vi "MHM_DLLDemo.vi"() -> ()   [LabVIEW 2019]
uses:
  enums/MHM_ConfigDataEnum.ctl
  enums/MHM_InterfaceEnum.ctl
  enums/MHM_ParamEnum.ctl
  enums/MHM_WriteVerifyEnum.ctl
  enums/EdsParamEnum.ctl
  enums/MHM_E2PRangeEnum.ctl
  enums/MHM_CalDataEnum.ctl
  enums/MHM_CalParamEnum.ctl
  enums/MHM_ErrorTypeEnum.ctl
  enums/MHM_CalCfgEnum.ctl
  enums/MHM_InterfaceInfoEnum.ctl
  MHM_1SL_interface.lvlib
panel:
  in  "StopButton":bool
  out "running":bool
  in  "TabControl":T1(tab)
  in  "MHM_InterfaceInfoEnum":T2
  out "MHM_InterfaceEnum":T3
  in  "MHM_InterfaceEnum":T3
  out "InterfaceLED":bool
  out "OpenLED":bool
  in  "MHM_Close":bool
  in  "MHM_GetInterface":bool
  in  "MHM_SetInterface":bool
  in  "MHM_Open":bool
  in  "pcInterfaceOption":string
  in  "MHM_GetInterfaceInfo":bool
  out "pcInterfaceInfo":string
  in  "MHM_Initialize":bool
  out "pulValue":u32 format="0x%02x"
  in  "ulValue":u32 format="0x%02x"
  in  "MHM_ConfigEnum":T4
  in  "MHM_ConfigEnum":T4
  in  "MHM_GetConfig":bool
  in  "MHM_SetConfig":bool
  in  "MHM_SwitchToBiSS":bool
  out "pulEnSsi":u32 format="0x%02x"
  in  "MHM_E2PRangeEnum":T5
  in  "MHM_WriteEeprom":bool
  in  "MHM_ReadStatusRegister":bool
  in  "ulWriteVerify":u32 format="0x%02x"
  in  "ulValue SetParam":u32 caption="ulValue" format="0x%02x"
  out "ulValue GetParam":u32 caption="pulValue" format="0x%02x"
  in  "MHM_WriteVerifyEnum":T6
  in  "MHM_ParamEnum":T7
  in  "MHM_ParamEnum":T7
  in  "MHM_WriteParams":bool
  in  "MHM_SetParam":bool
  in  "MHM_GetParam":bool
  in  "MHM_ReadParams":bool
  in  "MHM_ReadEeprom":bool
  in  "MHM_E2PRangeEnum":T5
  out "pulValid":u32[](array[numeric]) format="0x%02x"
  in  "MHM_GetCorrectedRegisters":bool
  out "pulCorrected":u32[](array[numeric]) format="0x%02x"
  in  "MHM_ReadGainRegister":bool
  in  "MHM_ReadSens":bool
  out "pulGain":u32 format="0x%02x"
  out "pSensorDataStruct":T8 {"pulGainRegister" format="0x%02x"; "pulPortRegister" format="0x%02x"; "pulStatusRegister" format="0x%02x"; "pulLifecounter" format="0x%02x"; "pulWarning" format="0x%02x"; "pulError" format="0x%02x"; "pulSingleturn" format="0x%02x"; "pulMultiturn" format="0x%02x"; "pulDataLength" format="0x%02x"; "pulLowData" format="0x%02x"; "pulHighData" format="0x%02x"}
  in  "MHM_CalParamEnum":T9
  in  "pulNumberOfBytes":u32 format="0x%02x"
  in  "ulCycles":u32=4096 format="0x%02x"
  in  "MHM_FullAcquisition":bool
  in  "ulCycles":u32=4096 format="0x%02x"
  in  "MHM_FullCalibration":bool
  in  "MHM_GetCalData":bool
  in  "MHM_GetCalParam":bool
  in  "MHM_CalDataEnum":T10
  out "plData":i32[](array[numeric]) format="0x%02x"
  out "plData":i32 format="0x%02x"
  in  "MHM_SetCalCfg":bool
  in  "MHM_CalCfgEnum":T11
  in  "lValue":i32 format="0x%02x"
  in  "MHM_CalCfgEnum":T11
  in  "MHM_GetCalCfg":bool
  out "plValue":i32 format="0x%02x"
  in  "MHM_SetCalData":bool
  in  "ulNumberOfBytes":u32 format="0x%02x"
  in  "MHM_CalDataEnum":T10
  in  "plData":i32[](array[numeric]) format="0x%02x"
  in  "MHM_AdjustGain":bool
  in  "MHM_ActivateCalCfg":bool
  in  "MHM_AcquireEx":bool
  in  "ulCycles":u32 format="0x%02x"
  in  "MHM_DeactivateCalCfg":bool
  in  "MHM_AnalyzeData":bool
  in  "MHM_Adjust":bool
  in  "MHM_WriteVerifyEnum":T6
  out "pulValue 2":u32 caption="pulValue" format="0x%02x"
  in  "ulValue":u32 format="0x%02x"
  in  "EdsParamEnum":T12 caption="MHM_EdsParamEnum"
  in  "MHM_EdsParamEnum":T12
  in  "MHM_SetEdsParam":bool
  in  "MHM_GetEdsParam":bool
  in  "MHM_ReadEdsParams":bool
  in  "MHM_UpdateEds":bool
  in  "ulCommand":u32=1 min=1 max=2 format="0x%02x"
  in  "MHM_ReadPorts":bool
  in  "MHM_WritePorts":bool
  in  "MHM_WriteCommand":bool
  in  "MHM_SPIActivate":bool
  in  "MHM_GetDLLVersion":bool
  in  "MHM_SaveParams":bool
  in  "MHM_LoadParams":bool
  in  "pcFilename":string
  in  "pcFilename":string
  out "pulDllVersion":u32[](array[numeric]) format="0x%02x"
  in  "ulPorts":u32 format="0x%02x"
  out "pulPorts":u32 format="0x%02x"
  in  "ulData":u32 format="0x%02x"
  in  "MHM_GetLastError":bool
  out "pulLastError":u32 format="0x%02x"
  out "MHM_ErrorTypeEnum":T13
  out "pcErrorText":string
  in  "MHM_Preset":bool
  in  "MHM_LoadRegister":bool
  in  "MHM_SaveRegister":bool
  in  "MHM_ReadRegister":bool
  in  "MHM_WriteRegister":bool
  in  "MHM_GetRegister":bool
  in  "MHM_SetRegister":bool
  in  "ulAdr":u32 format="0x%02x"
  in  "ulValue 2":u32 caption="ulValue" format="0x%02x"
  in  "MHM_WriteVerifyEnum 2":T6 caption="MHM_WriteVerifyEnum"
  in  "ulAdr":u32 format="0x%02x"
  out "pulValue":u32 format="0x%02x"
  in  "ulAdr 3":u32 caption="ulAdr" format="0x%02x"
  in  "pulNumberOfBytes":u32 format="0x%02x"
  in  "pulData":u32[](array[numeric]) format="0x%02x"
  out "pulData":u32[](array[numeric]) format="0x%02x"
  in  "pulNumberOfBytes":u32 format="0x%02x"
  in  "ulAdr":u32 format="0x%02x"
  in  "pcFilename 3":string caption="pcFilename"
  in  "ulAdr 5":u32 caption="ulAdr" format="0x%02x"
  in  "pulData 3":u32[](array[numeric]) caption="pulData" format="0x%02x"
  in  "pulNumberOfBytes5":u32 caption="pulNumberOfBytes" format="0x%02x"
  in  "pcFilename":string
  in  "ulAdr":u32 format="0x%02x"
  out "pulData":u32[](array[numeric]) format="0x%02x"
  in  "pulNumerOfBytes":u32 format="0x%02x"
  in  "MHM_WriteRegister_I2C":bool
  in  "ulAdr":u32 format="0x%02x"
  in  "ulNumberOfBytes":u32 format="0x%02x"
  in  "ulI2CSlaveAdr":u32 format="0x%02x"
  in  "pulData":u32[](array[numeric]) format="0x%02x"
  in  "MHM_ReadRegister_I2C":bool
  in  "ulAdr":u32 format="0x%02x"
  in  "pulNumberOfBytes":u32 format="0x%02x"
  in  "ulI2CSlaveAdr":u32 format="0x%02x"
  out "pulData":u32[](array[numeric]) format="0x%02x"
  in  "MHM_WriteRegister_I2C_EX":bool
  in  "ulArraySize":u32 format="0x%02x"
  in  "ulI2CSlaveAdr":u32 format="0x%02x"
  in  "pulData":u32[](array[numeric]) format="0x%02x"
  in  "pulValid":u32[](array[numeric]) format="0x%02x"
  in  "MHM_LoadRegister_EX":bool
  in  "pcFilename":string
  in  "ulArraySize":u32=256 format="0x%02x"
  out "pulData":u32[](array[numeric]) format="0x%02x"
  out "pulValid":u32[](array[numeric]) format="0x%02x"
  in  "MHM_SaveRegister_EX":bool
  in  "pcFilename":string
  in  "ulAdr":u32 format="0x%02x"
  in  "pulNumberOfBytes":u32 format="0x%02x"
  in  "pulData":u32[](array[numeric]) format="0x%02x"
  # "MHM_DLLDemo"
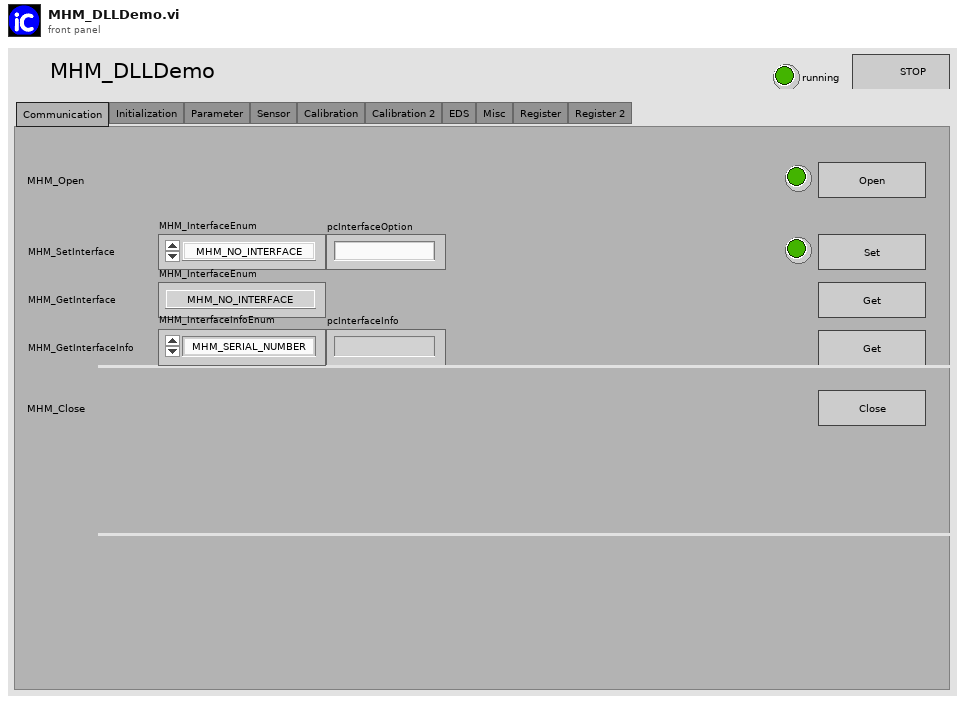
[diagram p1: front panel]
types:
  T1 = enum32{"Communication", "Initialization", "Parameter", "Sensor", "Calibration", "Calibration 2", "EDS", "Misc", "Register", "Register 2"}
  T2 = typedef "MHM_InterfaceInfoEnum.ctl" = enum16{"MHM_SERIAL_NUMBER"}
  T3 = typedef "MHM_InterfaceEnum.ctl" = enum16{"MHM_NO_INTERFACE", "MHM_MB3U_SPI", "MHM_MB3U_BISS", "MHM_MB4U", "MHM_MB5U"}
  T4 = typedef "MHM_ConfigDataEnum.ctl" = enum16{"MHM_CHIPVERSION", "MHM_USEUSB", "MHM_USELPT", "MHM_MASTERVER", "MHM_MASTERREV", "MHM_SLAVE_ID", "MHM_SLAVECOUNT", "MHM_FREQ_SCD", "MHM_FREQ_AGS", "MHM_FREQ_SPI", "MHM_CLKENI", "MHM_BP", "MHM_MT_TYPE", "MHM_RESERVED0", "MHM_RESERVED1", "MHM_RESERVED2", "MHM_RESERVED3", "MHM_FREQ_SSI", "MHM_READ_STATUS_ENABLE", "MHM_READ_PORTS_ENABLE", "MHM_READ_GAIN_ENABLE", "MHM_USB_PERFORMANCE", "MHM_ENABLE_TTL", "MHM_UPDATE_BISSID_ENABLE", "eMHM_DISABLE_AUTOMATIC_TTL_SWITCH"}
  T5 = typedef "MHM_E2PRangeEnum.ctl" = enum16{"MHM_E2P_CFG_MHM", "MHM_E2P_CFG_MT", "MHM_E2P_EDS", "MHM_E2P_ALL", "MHM_E2P_CFG_MHM_NO_OFFS"}
  T6 = typedef "MHM_WriteVerifyEnum.ctl" = enum16{"MHM_SETONLY", "MHM_WRITE", "MHM_VERIFY"}
  T7 = typedef "MHM_ParamEnum.ctl" = enum16{"MHM_AVGFILT", "MHM_TLF", "MHM_DIR", "MHM_HYS", "MHM_RESO_MT", "MHM_RESO_ST", "MHM_CF_MTI", "MHM_SBL_MTI", "MHM_EBL_MTI", "MHM_GET_MTI", "MHM_CFG_IOP", "MHM_MT12", "MHM_RTX_MODE", "MHM_BIN_SSI", "MHM_EXT_SSI", "MHM_ENSSI", "MHM_VOSS", "MHM_VOSC", "MHM_CIBM", "MHM_ENF", "MHM_TEST", "MHM_GAINF", "MHM_GAINR", "MHM_GCC", "MHM_ENAC", "MHM_CRCS", "MHM_ENLC", "MHM_REGPROT", "MHM_INSPROT", "MHM_PRES_IO1", "MHM_DIR_IO2", "MHM_ENCMD3", "MHM_ENCMD2", "MHM_CRC_CFG", "MHM_OFFS_MT", "MHM_OFFS_ST", "MHM_CRC_OFFS", "MHM_PSET_MT", "MHM_PSET_ST", "MHM_CRC_PSET", "MHM_ERR_CFG", "MHM_ERR_OFFS", "MHM_ERR_POS", "MHM_ERR_EXT", "MHM_ERR_AMIN", "MHM_ERR_AMAX", "MHM_ERR_MTI", "MHM_ERR_MT", "MHM_GAIN", "MHM_EDSBANK", "MHM_PRO_ID", "MHM_DEV_ID0", "MHM_DEV_ID1", "MHM_DEV_ID2", "MHM_DEV_ID3", "MHM_DEV_ID4", "MHM_DEV_ID5", "MHM_MFG_ID0", "MHM_MFG_ID1", "MHM_HARMCAL", "MHM_DISBISS", "MHM_NTOA", "MHM_ENCMD01", "MHM_CHIP_REL"}
  T8 = cluster{"pulHighData":u32, "pulLowData":u32, "pulDataLength":u32, "pulMultiturn":u32, "pulSingleturn":u32, "pulError":u32, "pulWarning":u32, "pulLifecounter":u32, "pulStatusRegister":u32, "pulPortRegister":u32, "pulGainRegister":u32}
  T9 = typedef "MHM_CalParamEnum.ctl" = enum16{"MHM_CAL_SINOFF", "MHM_CAL_COSOFF", "MHM_CAL_GAINCOSCORR", "MHM_CAL_HARM4", "MHM_CAL_RPM"}
  T10 = typedef "MHM_CalDataEnum.ctl" = enum16{"MHM_DUTRAW", "MHM_DUTCONT", "MHM_REFCONT", "MHM_DUTERR", "MHM_ADJERR", "MHM_REFRAW"}
  T11 = typedef "MHM_CalCfgEnum.ctl" = enum16{"MHM_CAL_FREQ_SPI", "MHM_CAL_FREQ_SCD", "MHM_CAL_FREQ_AGS", "MHM_CAL_REF_TYPE", "MHM_CAL_REF_RES", "MHM_CAL_REF_PER", "MHM_CAL_QUALITY_CHECK"}
  T12 = typedef "EdsParamEnum.ctl" = enum16{"EDS_EDS_VER", "EDS_EDS_LEN", "EDS_USR_STA", "EDS_USR_END", "EDS_TMA", "EDS_TO_MIN", "EDS_TO_MAX", "EDS_TOS_MIN", "EDS_TOS_MAX", "EDS_TCLK_MIN", "EDS_TCLK_MAX", "EDS_TCYC", "EDS_TBUSY_S", "EDS_BUSY_S", "EDS_PON_DLY", "EDS_DC_NUM", "EDS_SL_NUM", "EDS_SL_OFF", "EDS_BANK1", "EDS_DLEN1", "EDS_FORMAT1_STOP", "EDS_FORMAT1_ALIGN", "EDS_FORMAT1_TYPE", "EDS_CPOLY1", "EDS_BANK2", "EDS_DLEN2", "EDS_FORMAT2_STOP", "EDS_FORMAT2_ALIGN", "EDS_FORMAT2_TYPE", "EDS_CPOLY2", "EDS_BANK3", "EDS_DLEN3", "EDS_FORMAT3_STOP", "EDS_FORMAT3_ALIGN", "EDS_FORMAT3_TYPE", "EDS_CPOLY3", "EDS_BANK4", "EDS_DLEN4", "EDS_FORMAT4_STOP", "EDS_FORMAT4_ALIGN", "EDS_FORMAT4_TYPE", "EDS_CPOLY4", "EDS_BANK5", "EDS_DLEN5", "EDS_FORMAT5_STOP", "EDS_FORMAT5_ALIGN", "EDS_FORMAT5_TYPE", "EDS_CPOLY5", "EDS_BANK6", "EDS_DLEN6", "EDS_FORMAT6_STOP", "EDS_FORMAT6_ALIGN", "EDS_FORMAT6_TYPE", "EDS_CPOLY6", "EDS_BANK7", "EDS_DLEN7", "EDS_FORMAT7_STOP", "EDS_FORMAT7_ALIGN", "EDS_FORMAT7_TYPE", "EDS_CPOLY7", "EDS_BANK8", "EDS_DLEN8", "EDS_FORMAT8_STOP", "EDS_FORMAT8_ALIGN", "EDS_FORMAT8_TYPE", "EDS_CPOLY8", "EDS_BC_OFF", "EDS_BP_VER", "EDS_BP_LEN", "EDS_BP_ID", "EDS_FB1", "EDS_FB2", "EDS_PON_PDL", "EDS_EN_TYP", "EDS_POS_NUM", "EDS_MT_LEN", "EDS_MT_FMT", "EDS_CO_LEN", "EDS_CO_FMT", "EDS_FI_LEN", "EDS_FI_FMT", "EDS_MT_CNT", "EDS_SIP_CNT", "EDS_SIP_RES", "EDS_CPOLY", "EDS_CSTART", "EDS_ABS_ACU", "EDS_REL_ACU", "EDS_SPD_ACU", "EDS_HYST", "EDS_SPD_MAX", "EDS_ACC_MAX", "EDS_TMP_MIN", "EDS_TMP_MAX", "EDS_VLT_MIN", "EDS_VLT_MAX", "EDS_CUR_MAX"}
  T13 = typedef "MHM_ErrorTypeEnum.ctl" = enum16{"MHM_NONE", "MHM_HINT", "MHM_WARNING", "MHM_PROGRAMMING_ERROR", "MHM_OPERATING_ERROR", "MHM_COMMUNICATION_ERROR"}
  T14 = cluster{"ulHighData":u32, "ulLowData":u32, "ulDataLength":u32, "ulMultiturn":u32, "ulSingleturn":u32, "ulError":u32, "ulWarning":u32, "ulLifecounter":u32, "ulStatusRegister":u32, "ulPortRegister":u32, "ulGainRegister":u32}
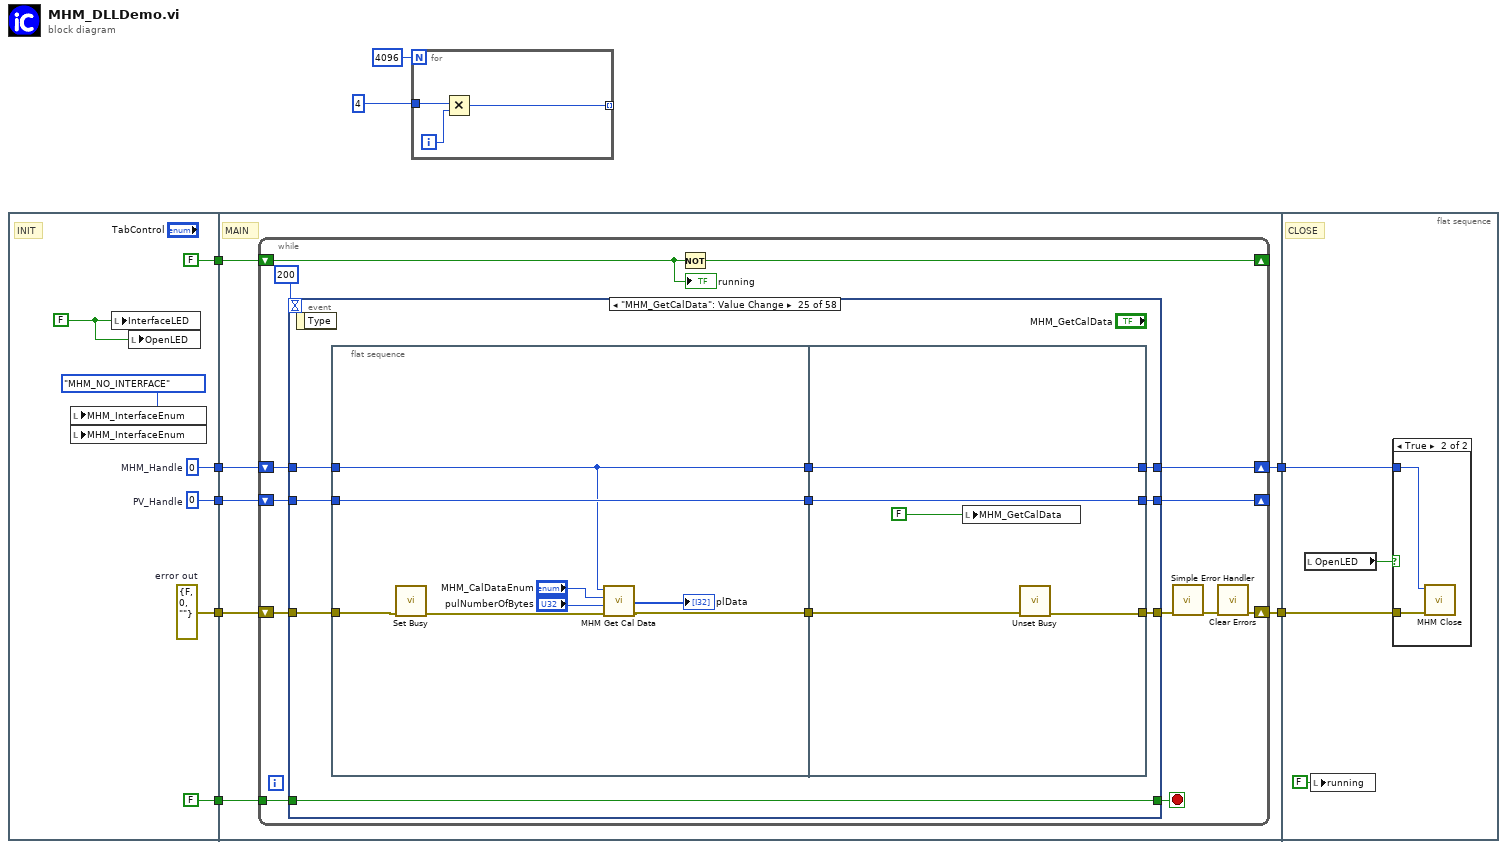
[diagram p0: block diagram]
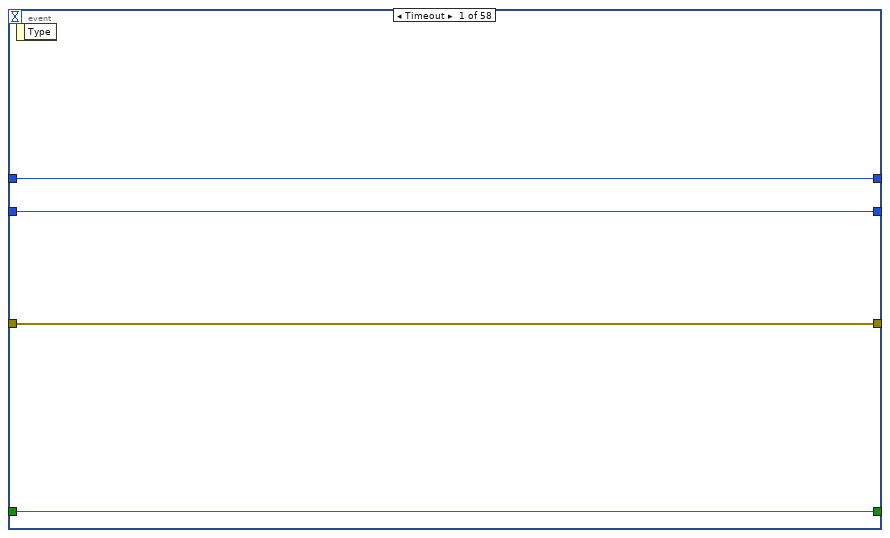
[diagram p2: hidden frame]
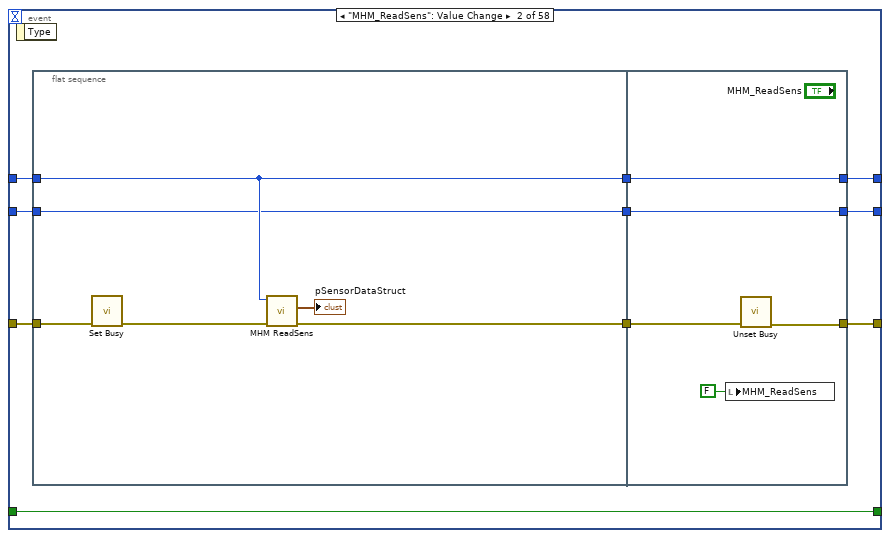
[diagram p3: hidden frame]
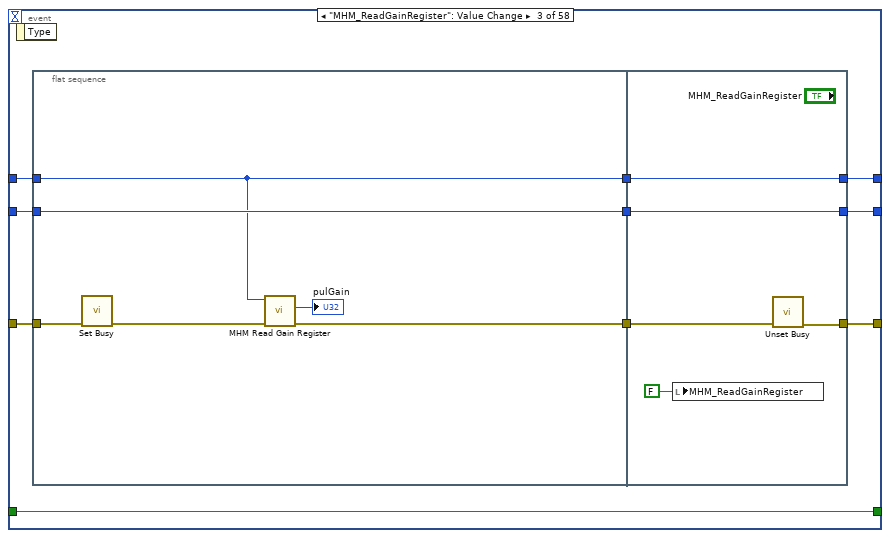
[diagram p4: hidden frame]
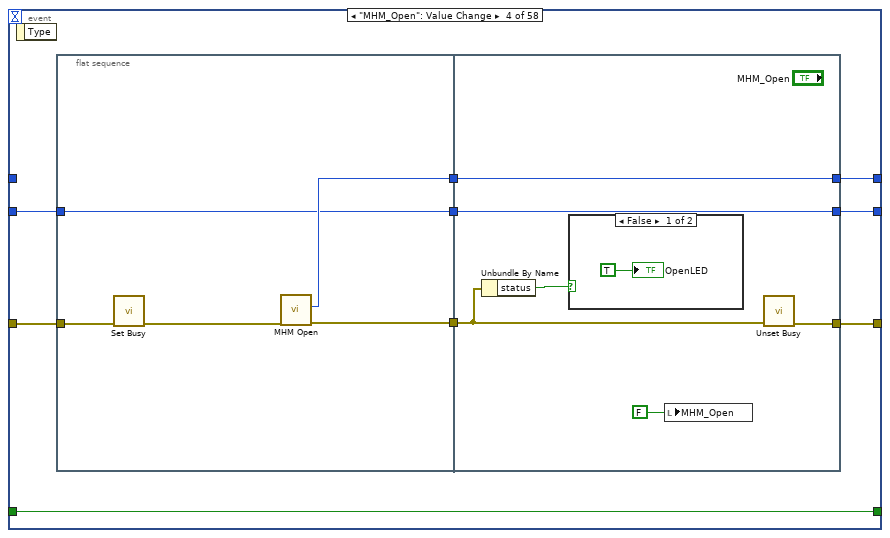
[diagram p5: hidden frame]
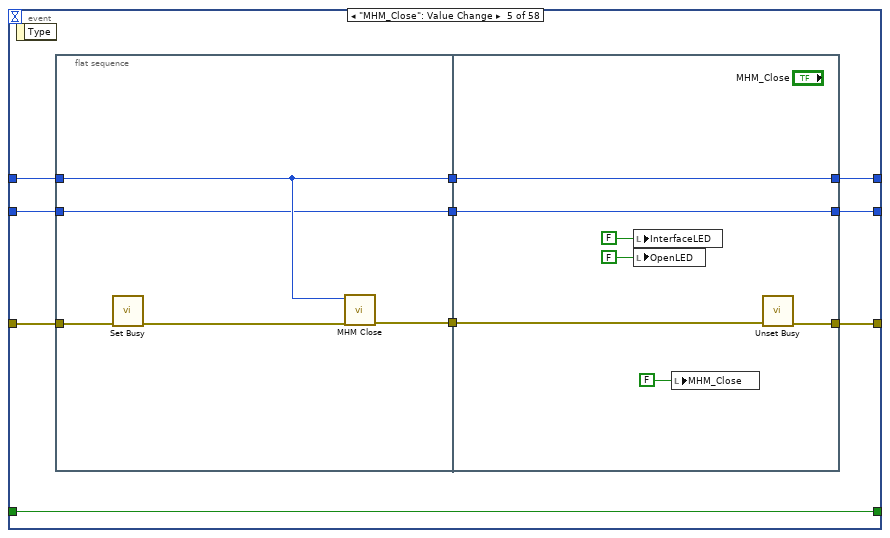
[diagram p7: hidden frame]
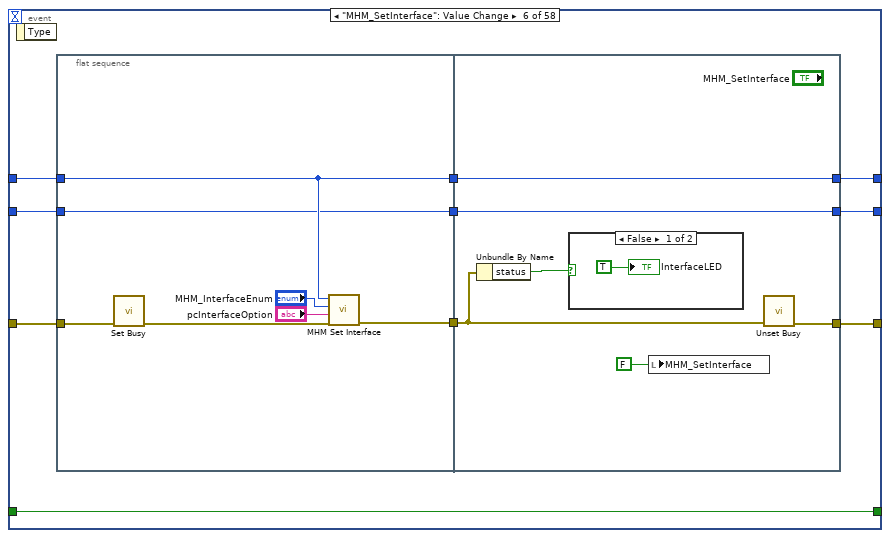
[diagram p8: hidden frame]
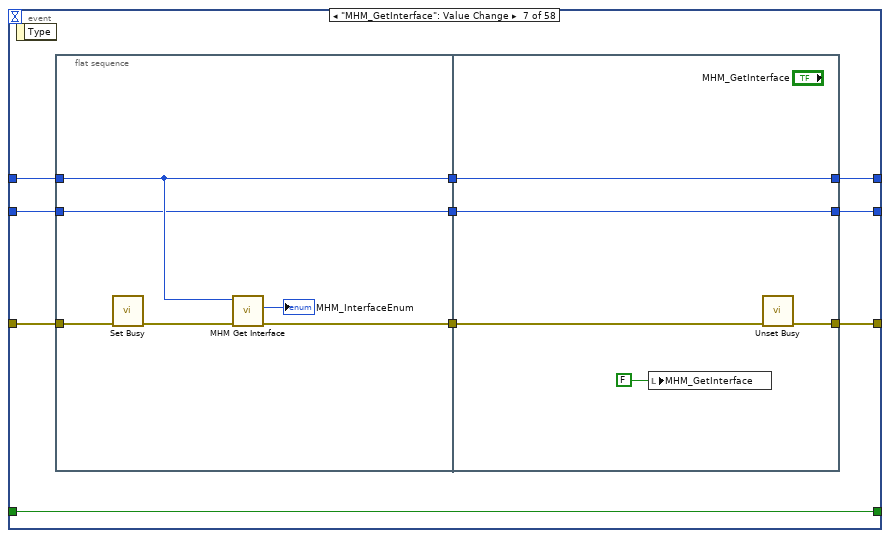
[diagram p10: hidden frame]
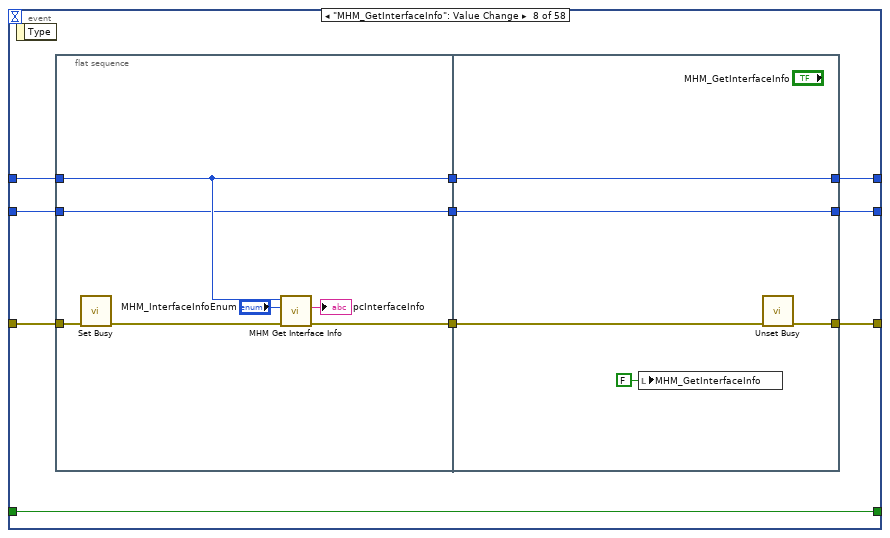
[diagram p11: hidden frame]
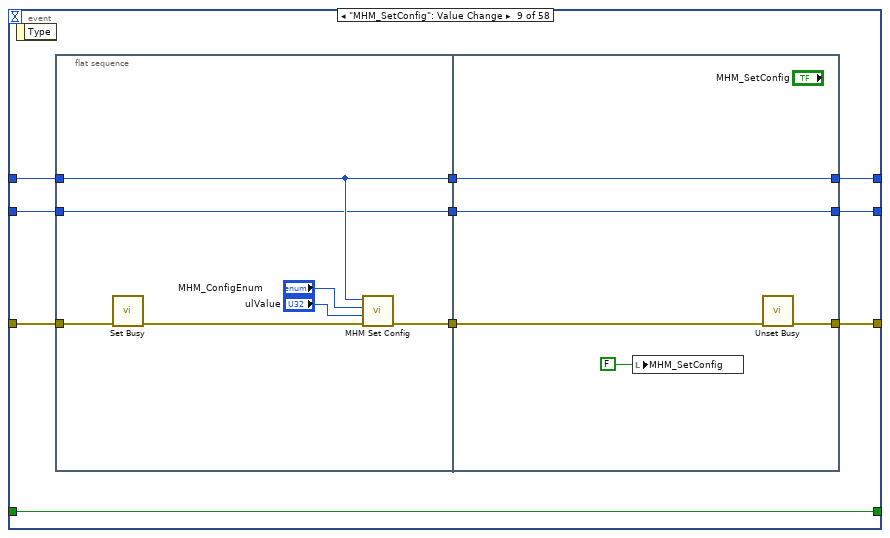
[diagram p12: hidden frame]
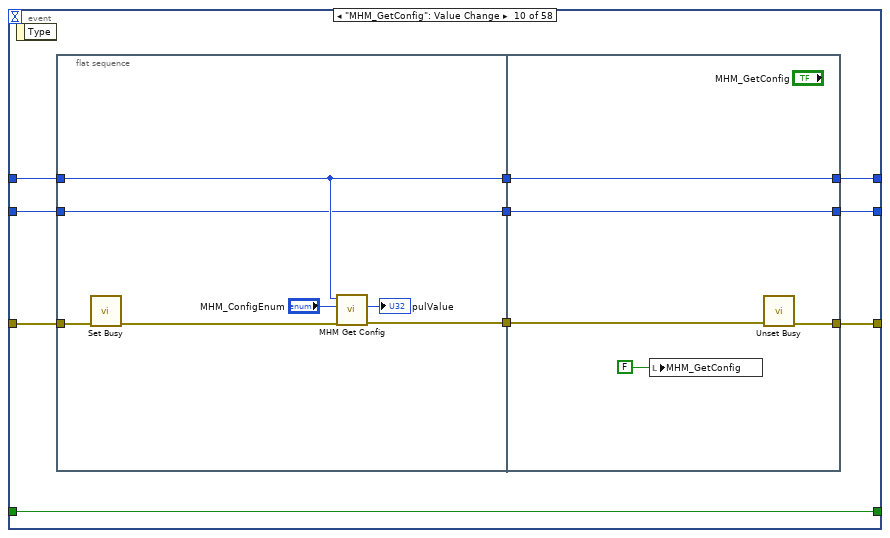
[diagram p13: hidden frame]
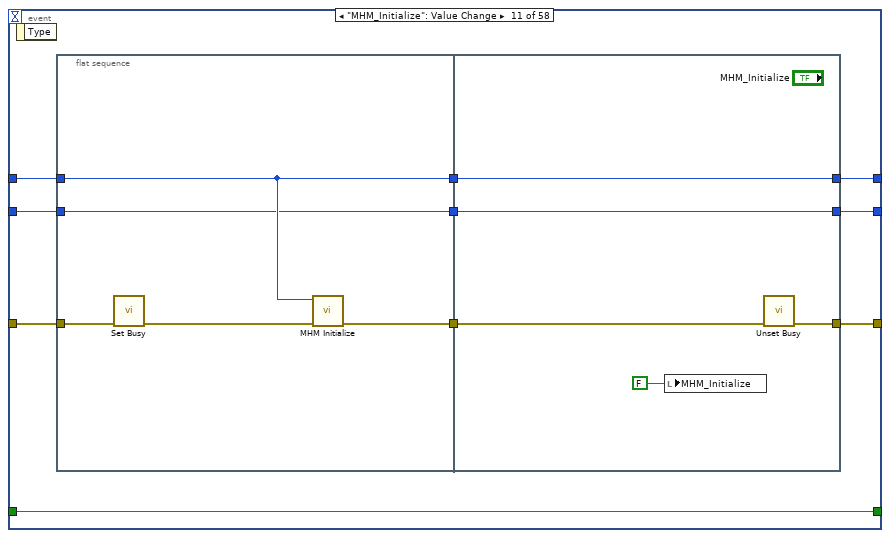
[diagram p14: hidden frame]
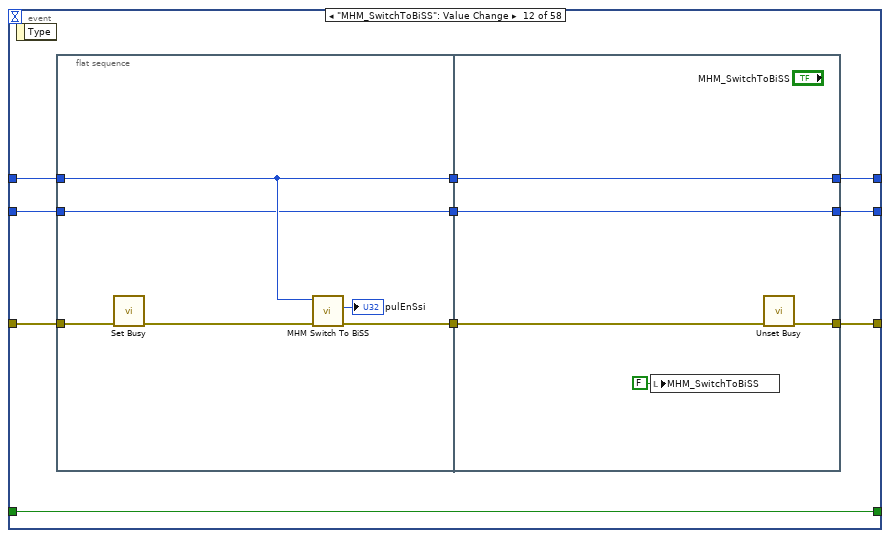
[diagram p15: hidden frame]
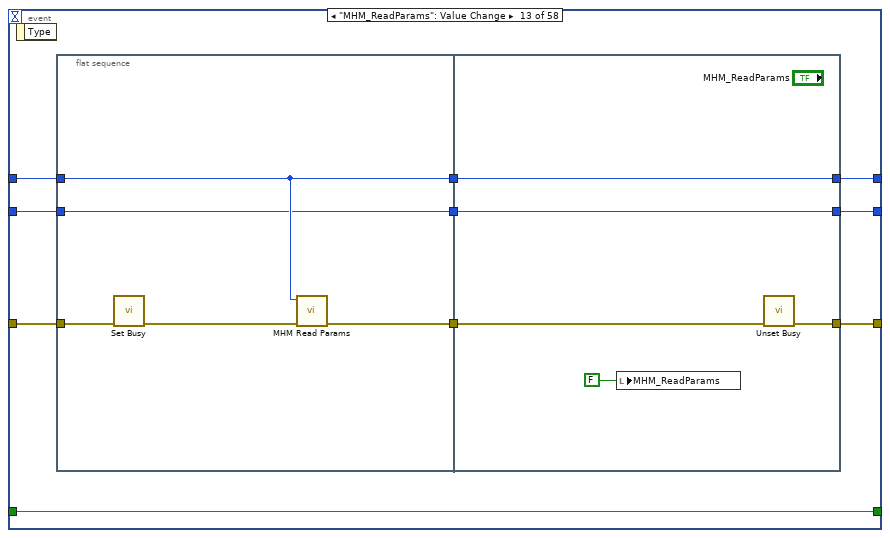
[diagram p16: hidden frame]
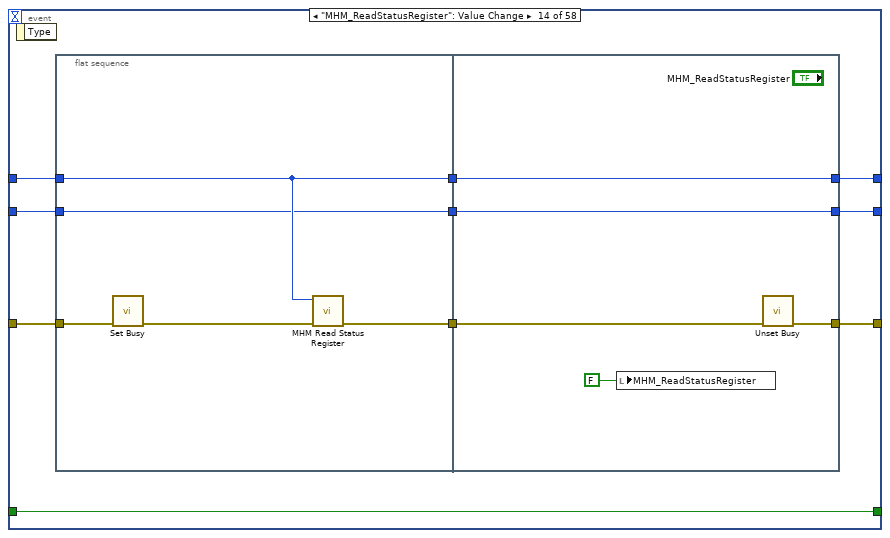
[diagram p17: hidden frame]
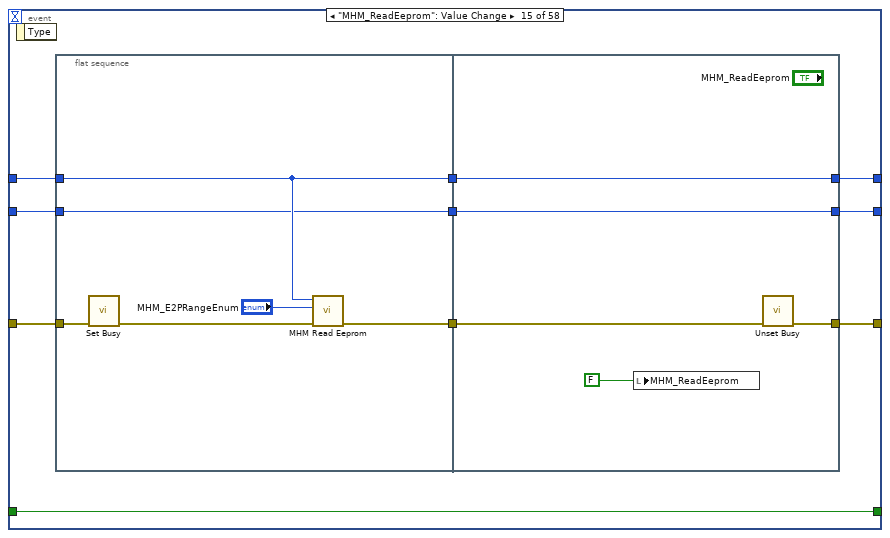
[diagram p18: hidden frame]
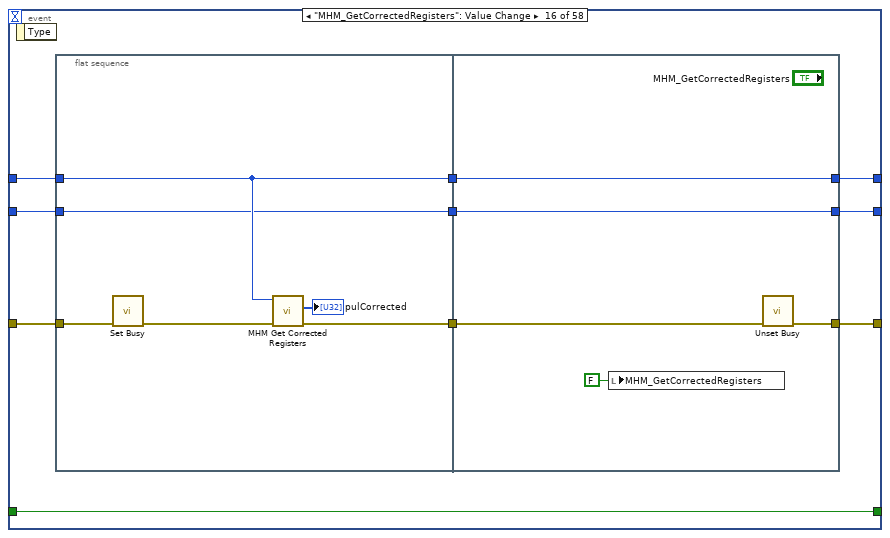
[diagram p19: hidden frame]
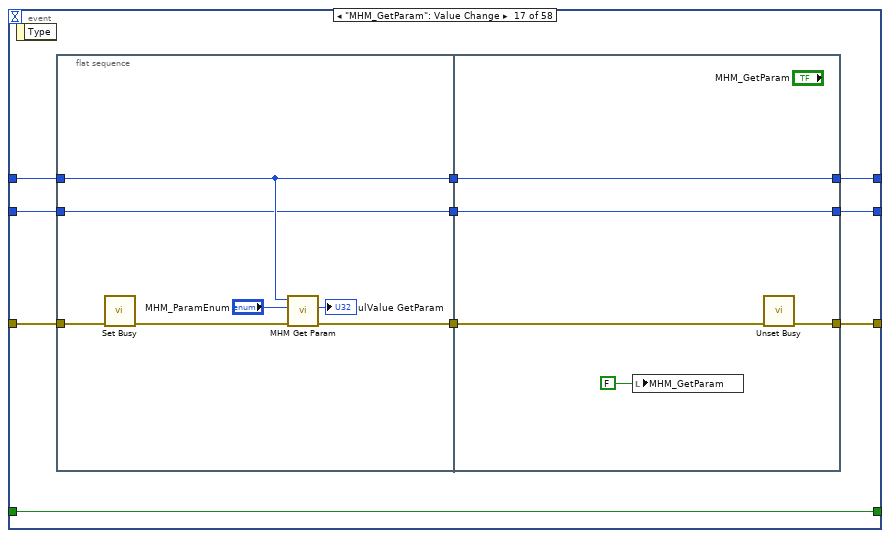
[diagram p20: hidden frame]
diagram:
  n1 = flat-sequence {
    tunnel: [FALSE] -> w9
    tunnel: [FALSE] -> w8
    tunnel: [w14] -> w7
    tunnel: [w13] -> w6
    tunnel: [w11] -> w3
    tunnel: w9 -> [w23]
    tunnel: w8 -> [w22]
    tunnel: w7 -> [w21]
    tunnel: w6 -> [w20]
    tunnel: [w19] -> w5
    tunnel: [w18] -> w4
    tunnel: w3 -> [w17]
    tunnel: w5 -> [w1263]
    tunnel: w4 -> [w1262]
    frame #0 {
      w11 = u32 0  # PV_Handle
      w12 = MHM_InterfaceEnum."MHM_NO_INTERFACE" ("MHM_InterfaceEnum")
      w10 = FALSE ("InterfaceLED")
      w13 = errorcluster {"status"=FALSE, "code"=0, "source"=""}  # error out
      w14 = u32 0  # MHM_Handle
      # "INIT"
      n2 = local write "MHM_InterfaceEnum"(w12) -> ()
      n3 = local write "MHM_InterfaceEnum"(w12) -> ()
      n4 = local write "InterfaceLED"(w10) -> ()
      n5 = local write "OpenLED"(w10) -> ()
    }
    frame #1 {
      # "MAIN"
      n6 = while {
        shift-right: [w36] -> _
        shift-left: w23 -> [w35]
        tunnel: w22 -> [w34]
        shift-right: [w27] -> w18
        shift-left: w21 -> [w32]
        shift-right: [w30] -> w19
        shift-left: w20 -> [w31]
        shift-right: [w25] -> _
        shift-left: w17 -> [w24]
        stop <- w33 stop-if-true
        n7 = event shown="[24] \"MHM_GetCalData\": Value Change" {
          selector: _ -> [_ _ _ _ _ _ _ _ _ _ _ _ _ _ _ _ _ _ _ _ _ _ _ _ _ _ _ _ _ _ _ _ _ _ _ _ _ _ _ _ _ _ _ _ _ _ _ _ _ _ _ _ _ _ _ _ _ _]
          dyn-events: _ -> [_ _ _ _ _ _ _ _ _ _ _ _ _ _ _ _ _ _ _ _ _ _ _ _ _ _ _ _ _ _ _ _ _ _ _ _ _ _ _ _ _ _ _ _ _ _ _ _ _ _ _ _ _ _ _ _ _ _]
          timeout: 200 -> [_ _ _ _ _ _ _ _ _ _ _ _ _ _ _ _ _ _ _ _ _ _ _ _ _ _ _ _ _ _ _ _ _ _ _ _ _ _ _ _ _ _ _ _ _ _ _ _ _ _ _ _ _ _ _ _ _ _]
          tunnel: w34 -> [w40 w41 w62 w91 w107 w135 w158 w179 w196 w223 w240 w260 w286 w305 w325 w346 w365 w385 w408 w436 w448 w470 w492 w513 w534 w557 w580 w602 w622 w642 w663 w683 w703 w733 w753 w775 w795 w816 w837 w855 w873 w895 w915 w939 w961 w982 w1001 w1029 w1050 w1074 w1092 w1116 w1140 w1164 w1188 w1212 w1236 w1261]
          tunnel: [w40 w41 w62 w91 w107 w135 w158 w179 w196 w223 w240 w260 w286 w305 w325 w346 w365 w385 w408 w436 w448 w470 w492 w513 w534 w557 w580 w602 w622 w642 w663 w683 w703 w733 w753 w775 w795 w816 w837 w855 w873 w895 w915 w939 w961 w982 w1001 w1029 w1050 w1074 w1092 w1116 w1140 w1164 w1188 w1212 w1236 w1260] -> w33
          tunnel: w32 -> [w39 w47 w68 _ w110 w132 w155 w176 w199 w221 w243 w263 w283 w303 w323 w344 w367 w389 w412 w434 w454 w476 w498 w519 w540 w563 w586 w608 w628 w648 w669 w689 w709 w731 w751 w773 w793 w813 w834 w854 w876 w898 w918 w937 w959 w980 w1004 w1027 w1048 w1071 w1095 w1119 w1143 w1167 w1191 w1215 w1239 w1258]
          tunnel: w31 -> [w37 w45 w66 w89 w113 w133 w157 w178 w201 w222 w246 w266 w285 w306 w326 w347 w368 w390 w413 w435 w452 w474 w496 w517 w538 w561 w584 w606 w626 w646 w667 w687 w707 w732 w752 w774 w794 w815 w836 w858 w878 w900 w920 w941 w962 w983 w1006 w1028 w1051 w1073 w1097 w1121 w1145 w1169 w1193 w1217 w1241 w1259]
          tunnel: [w37 w42 w63 w90 w112 w134 w159 w180 w202 w224 w245 w265 w287 w307 w327 w348 w369 w391 w414 w432 w449 w471 w493 w514 w535 w558 w581 w603 w623 w643 w664 w684 w704 w724 w749 w771 w786 w817 w838 w856 w879 w894 w921 w942 w963 w984 w1007 w1030 w1052 w1075 w1098 w1122 w1146 w1170 w1194 w1218 w1242 w1259] -> w28
          tunnel: [w39 w44 w65 w86 w108 w129 w153 w174 w197 w218 w241 w261 w281 w301 w321 w342 w363 w386 w409 w430 w450 w472 w494 w515 w536 w559 w582 w604 w624 w644 w665 w685 w705 w729 w747 w769 w791 w811 w832 w852 w874 w896 w916 w936 w957 w978 w1002 w1025 w1046 w1069 w1093 w1117 w1141 w1165 w1189 w1213 w1237 w1258] -> w27
          tunnel: [w38 w43 w64 w83 w104 w126 w150 w171 w193 w215 w237 w257 w278 w298 w318 w339 w360 w382 w405 w427 w451 w473 w495 w516 w537 w560 w583 w605 w625 w645 w666 w686 w706 w726 w744 w766 w788 w808 w829 w849 w870 w891 w912 w933 w954 w975 w998 w1021 w1043 w1066 w1089 w1113 w1137 w1161 w1185 w1209 w1233 w1257] -> w25
          tunnel: w24 -> [w38 w46 w67 w84 w105 w127 w151 w172 w194 w216 w238 w258 w279 w299 w319 w340 w361 w383 w406 w428 w453 w475 w497 w518 w539 w562 w585 w607 w627 w647 w668 w688 w708 w727 w745 w767 w789 w809 w830 w850 w871 w892 w913 w934 w955 w976 w999 w1022 w1044 w1067 w1090 w1114 w1138 w1162 w1186 w1210 w1234 w1257]
          event Timeout {
            n8 = event-data() -> ()  [unwired: 2 out]
          }
          event "MHM_ReadSens": Value Change {
            n9 = event-data() -> ()  [unwired: 2 out]
            n10 = flat-sequence {
              tunnel: [w56] -> w50
              tunnel: w47 -> [w56]
              tunnel: w45 -> [w52]
              tunnel: [w53] -> w49
              tunnel: w46 -> [w55]
              tunnel: [w55] -> w48
              tunnel: w50 -> [w61]
              tunnel: [w61] -> w44
              tunnel: w49 -> [w58]
              tunnel: [w57] -> w42
              tunnel: w48 -> [w59]
              tunnel: [w59] -> w43
              frame #0 {
                n11 = call <vilib>:"Set Busy.vi"("error in (no error)"=w52) -> ("error out"=w51:errorcluster)  [unwired: 3 in, 7 out]
                n12 = call "MHM ReadSens.vi"("error in (no error)"=w51, "ulMHMHandle"=w56) -> ("error out"=w53:errorcluster, "pSensorDataStruct"=→"pSensorDataStruct":T14)  [unwired: 7 in, 1 out]
              }
              frame #1 {
                n13 = local write "MHM_ReadSens"(FALSE ("MHM_ReadSensor")) -> ()
                n14 = call <vilib>:"Unset Busy.vi"("error in (no error)"=w58) -> ("error out"=w57:errorcluster)  [unwired: 1 in, 9 out]
              }
            }
          }
          event "MHM_ReadGainRegister": Value Change {
            n15 = event-data() -> ()  [unwired: 2 out]
            n16 = flat-sequence {
              tunnel: [w74] -> w71
              tunnel: w68 -> [w74]
              tunnel: w66 -> [w73]
              tunnel: [w75] -> w70
              tunnel: w67 -> [w77]
              tunnel: [w77] -> w69
              tunnel: w71 -> [w82]
              tunnel: [w82] -> w65
              tunnel: w70 -> [w79]
              tunnel: [w78] -> w63
              tunnel: w69 -> [w80]
              tunnel: [w80] -> w64
              frame #0 {
                n17 = call <vilib>:"Set Busy.vi"("error in (no error)"=w73) -> ("error out"=w72:errorcluster)  [unwired: 3 in, 7 out]
                n18 = call "MHM Read Gain Register.vi"("error in (no error)"=w72, "ulMHMHandle"=w74) -> ("error out"=w75:errorcluster, "pulGain"=→"pulGain":u32)  [unwired: 7 in, 1 out]
              }
              frame #1 {
                n19 = local write "MHM_ReadGainRegister"(FALSE ("MHM_ReadSensor")) -> ()
                n20 = call <vilib>:"Unset Busy.vi"("error in (no error)"=w79) -> ("error out"=w78:errorcluster)  [unwired: 1 in, 9 out]
              }
            }
          }
          event "MHM_Open": Value Change {
            n21 = event-data() -> ()  [unwired: 2 out]
            n22 = flat-sequence {
              tunnel: w89 -> [w96]
              tunnel: [w94] -> w88
              tunnel: [w93] -> w87
              tunnel: [w92] -> w85
              tunnel: w84 -> [w92]
              tunnel: [w102] -> w90
              tunnel: w88 -> [w99]
              tunnel: [w101] -> w86
              tunnel: w87 -> [w101]
              tunnel: w85 -> [w97]
              tunnel: [w97] -> w83
              frame #0 {
                n23 = call <vilib>:"Set Busy.vi"("error in (no error)"=w96) -> ("error out"=w95:errorcluster)  [unwired: 3 in, 7 out]
                n24 = call "MHM Open.vi"("error in (no error)"=w95) -> ("error out"=w94:errorcluster, "pulMHMHandle"=w93:u32)  [unwired: 8 in, 1 out]
              }
              frame #1 {
                n25 = Unbundle By Name(w99) -> ("status"=w98:bool)
                n26 = case shown="False" w98 {
                  frame False {
                    "OpenLED" <- TRUE ("OpenLED")
                  }
                  frame True {
                  }
                }
                n27 = local write "MHM_Open"(FALSE ("MHM_Open")) -> ()
                n28 = call <vilib>:"Unset Busy.vi"("error in (no error)"=w99) -> ("error out"=w102:errorcluster)  [unwired: 1 in, 9 out]
              }
            }
          }
          event "MHM_Close": Value Change {
            n29 = event-data() -> ()  [unwired: 2 out]
            n30 = flat-sequence {
              tunnel: w113 -> [w118]
              tunnel: [w116] -> w111
              tunnel: w110 -> [w115]
              tunnel: [w115] -> w109
              tunnel: [w114] -> w106
              tunnel: w105 -> [w114]
              tunnel: [w125] -> w112
              tunnel: w111 -> [w122]
              tunnel: [w124] -> w108
              tunnel: w109 -> [w124]
              tunnel: w106 -> [w119]
              tunnel: [w119] -> w104
              frame #0 {
                n31 = call <vilib>:"Set Busy.vi"("error in (no error)"=w118) -> ("error out"=w117:errorcluster)  [unwired: 3 in, 7 out]
                n32 = call "MHM Close.vi"("error in (no error)"=w117, "ulMHMHandle"=w115) -> ("error out"=w116:errorcluster)  [unwired: 8 in, 1 out]
              }
              frame #1 {
                n33 = local write "InterfaceLED"(FALSE ("InterfaceLED")) -> ()
                n34 = local write "OpenLED"(FALSE ("OpenLED")) -> ()
                n35 = local write "MHM_Close"(FALSE ("MHM_Close")) -> ()
                n36 = call <vilib>:"Unset Busy.vi"("error in (no error)"=w122) -> ("error out"=w125:errorcluster)  [unwired: 1 in, 9 out]
              }
            }
          }
          event "MHM_SetInterface": Value Change {
            n37 = event-data() -> ()  [unwired: 2 out]
            n38 = flat-sequence {
              tunnel: w133 -> [w142]
              tunnel: w132 -> [w138]
              tunnel: [w139] -> w131
              tunnel: [w138] -> w130
              tunnel: [w136] -> w128
              tunnel: w127 -> [w136]
              tunnel: [w148] -> w134
              tunnel: w131 -> [w146]
              tunnel: [w147] -> w129
              tunnel: w130 -> [w147]
              tunnel: w128 -> [w143]
              tunnel: [w143] -> w126
              frame #0 {
                n39 = call <vilib>:"Set Busy.vi"("error in (no error)"=w142) -> ("error out"=w141:errorcluster)  [unwired: 3 in, 7 out]
                n40 = call "MHM Set Interface.vi"("error in (no error)"=w141, "pcInterfaceOption"="pcInterfaceOption", "ulInterface"="MHM_InterfaceEnum", "ulMHMHandle"=w138) -> ("error out"=w139:errorcluster)  [unwired: 6 in, 1 out]
              }
              frame #1 {
                n41 = Unbundle By Name(w146) -> ("status"=w145:bool)
                n42 = case shown="False" w145 {
                  frame False {
                    "InterfaceLED" <- TRUE ("InterfaceLED")
                  }
                  frame True {
                  }
                }
                n43 = local write "MHM_SetInterface"(FALSE ("MHM_SetInterface")) -> ()
                n44 = call <vilib>:"Unset Busy.vi"("error in (no error)"=w146) -> ("error out"=w148:errorcluster)  [unwired: 1 in, 9 out]
              }
            }
          }
          event "MHM_GetInterface": Value Change {
            n45 = event-data() -> ()  [unwired: 2 out]
            n46 = flat-sequence {
              tunnel: w157 -> [w165]
              tunnel: [w163] -> w156
              tunnel: w155 -> [w161]
              tunnel: [w161] -> w154
              tunnel: [w160] -> w152
              tunnel: w151 -> [w160]
              tunnel: [w170] -> w159
              tunnel: w156 -> [w169]
              tunnel: w154 -> [w168]
              tunnel: [w168] -> w153
              tunnel: w152 -> [w166]
              tunnel: [w166] -> w150
              frame #0 {
                n47 = call <vilib>:"Set Busy.vi"("error in (no error)"=w165) -> ("error out"=w164:errorcluster)  [unwired: 3 in, 7 out]
                n48 = call "MHM Get Interface.vi"("error in (no error)"=w164, "ulMHMHandle"=w161) -> ("error out"=w163:errorcluster, "pulInterface"=→"MHM_InterfaceEnum":u32)  [unwired: 7 in, 1 out]
              }
              frame #1 {
                n49 = local write "MHM_GetInterface"(FALSE ("MHM_GetInterface")) -> ()
                n50 = call <vilib>:"Unset Busy.vi"("error in (no error)"=w169) -> ("error out"=w170:errorcluster)  [unwired: 1 in, 9 out]
              }
            }
          }
          event "MHM_GetInterfaceInfo": Value Change {
            n51 = event-data() -> ()  [unwired: 2 out]
            n52 = flat-sequence {
              tunnel: w178 -> [w187]
              tunnel: [w185] -> w177
              tunnel: w176 -> [w184]
              tunnel: [w184] -> w175
              tunnel: [w183] -> w173
              tunnel: w172 -> [w183]
              tunnel: [w192] -> w180
              tunnel: w177 -> [w191]
              tunnel: w175 -> [w190]
              tunnel: [w190] -> w174
              tunnel: w173 -> [w188]
              tunnel: [w188] -> w171
              frame #0 {
                n53 = call <vilib>:"Set Busy.vi"("error in (no error)"=w187) -> ("error out"=w186:errorcluster)  [unwired: 3 in, 7 out]
                n54 = call "MHM Get Interface Info.vi"("error in (no error)"=w186, "ulIndex"="MHM_InterfaceInfoEnum", "ulMHMHandle"=w184) -> ("error out"=w185:errorcluster, "pcInterfaceInfo"=→"pcInterfaceInfo":string)  [unwired: 6 in, 1 out]
              }
              frame #1 {
                n55 = local write "MHM_GetInterfaceInfo"(FALSE ("MHM_GetInterface")) -> ()
                n56 = call <vilib>:"Unset Busy.vi"("error in (no error)"=w191) -> ("error out"=w192:errorcluster)  [unwired: 1 in, 9 out]
              }
            }
          }
          event "MHM_SetConfig": Value Change {
            n57 = event-data() -> ()  [unwired: 2 out]
            n58 = flat-sequence {
              tunnel: w201 -> [w209]
              tunnel: [w207] -> w200
              tunnel: w199 -> [w206]
              tunnel: [w206] -> w198
              tunnel: [w203] -> w195
              tunnel: w194 -> [w203]
              tunnel: [w214] -> w202
              tunnel: w200 -> [w213]
              tunnel: [w212] -> w197
              tunnel: w198 -> [w212]
              tunnel: w195 -> [w210]
              tunnel: [w210] -> w193
              frame #0 {
                n59 = call <vilib>:"Set Busy.vi"("error in (no error)"=w209) -> ("error out"=w208:errorcluster)  [unwired: 3 in, 7 out]
                n60 = call "MHM Set Config.vi"("error in (no error)"=w208, "ulValue"="ulValue", "ulConfig"="MHM_ConfigEnum", "ulMHMHandle"=w206) -> ("error out"=w207:errorcluster)  [unwired: 6 in, 1 out]
              }
              frame #1 {
                n61 = local write "MHM_SetConfig"(FALSE ("MHM_SetConfig")) -> ()
                n62 = call <vilib>:"Unset Busy.vi"("error in (no error)"=w213) -> ("error out"=w214:errorcluster)  [unwired: 1 in, 9 out]
              }
            }
          }
          event "MHM_GetConfig": Value Change {
            n63 = event-data() -> ()  [unwired: 2 out]
            n64 = flat-sequence {
              tunnel: w222 -> [w231]
              tunnel: w221 -> [w226]
              tunnel: [w229] -> w220
              tunnel: [w226] -> w219
              tunnel: [w225] -> w217
              tunnel: w216 -> [w225]
              tunnel: [w236] -> w224
              tunnel: w220 -> [w235]
              tunnel: [w234] -> w218
              tunnel: w219 -> [w234]
              tunnel: w217 -> [w232]
              tunnel: [w232] -> w215
              frame #0 {
                n65 = call <vilib>:"Set Busy.vi"("error in (no error)"=w231) -> ("error out"=w230:errorcluster)  [unwired: 3 in, 7 out]
                n66 = call "MHM Get Config.vi"("error in (no error)"=w230, "ulConfig"="MHM_ConfigEnum", "ulMHMHandle"=w226) -> ("error out"=w229:errorcluster, "pulValue"=→"pulValue":u32)  [unwired: 6 in, 1 out]
              }
              frame #1 {
                n67 = local write "MHM_GetConfig"(FALSE ("MHM_GetConfig")) -> ()
                n68 = call <vilib>:"Unset Busy.vi"("error in (no error)"=w235) -> ("error out"=w236:errorcluster)  [unwired: 1 in, 9 out]
              }
            }
          }
          event "MHM_Initialize": Value Change {
            n69 = event-data() -> ()  [unwired: 2 out]
            n70 = flat-sequence {
              tunnel: w246 -> [w251]
              tunnel: [w249] -> w244
              tunnel: w243 -> [w248]
              tunnel: [w248] -> w242
              tunnel: [w247] -> w239
              tunnel: w238 -> [w247]
              tunnel: [w256] -> w245
              tunnel: w244 -> [w255]
              tunnel: [w254] -> w241
              tunnel: w242 -> [w254]
              tunnel: w239 -> [w252]
              tunnel: [w252] -> w237
              frame #0 {
                n71 = call <vilib>:"Set Busy.vi"("error in (no error)"=w251) -> ("error out"=w250:errorcluster)  [unwired: 3 in, 7 out]
                n72 = call "MHM Initialize.vi"("error in (no error)"=w250, "ulMHMHandle"=w248) -> ("error out"=w249:errorcluster)  [unwired: 8 in, 1 out]
              }
              frame #1 {
                n73 = local write "MHM_Initialize"(FALSE ("MHM_Initialize")) -> ()
                n74 = call <vilib>:"Unset Busy.vi"("error in (no error)"=w255) -> ("error out"=w256:errorcluster)  [unwired: 1 in, 9 out]
              }
            }
          }
          event "MHM_SwitchToBiSS": Value Change {
            n75 = event-data() -> ()  [unwired: 2 out]
            n76 = flat-sequence {
              tunnel: w266 -> [w272]
              tunnel: [w270] -> w264
              tunnel: w263 -> [w269]
              tunnel: [w269] -> w262
              tunnel: [w268] -> w259
              tunnel: w258 -> [w268]
              tunnel: [w277] -> w265
              tunnel: w264 -> [w276]
              tunnel: [w275] -> w261
              tunnel: w262 -> [w275]
              tunnel: w259 -> [w273]
              tunnel: [w273] -> w257
              frame #0 {
                n77 = call <vilib>:"Set Busy.vi"("error in (no error)"=w272) -> ("error out"=w271:errorcluster)  [unwired: 3 in, 7 out]
                n78 = call "MHM Switch To BiSS.vi"("error in (no error)"=w271, "ulMHMHandle"=w269) -> ("error out"=w270:errorcluster, "pulEnSsi"=→"pulEnSsi":u32)  [unwired: 7 in, 1 out]
              }
              frame #1 {
                n79 = local write "MHM_SwitchToBiSS"(FALSE ("MHM_Initialize")) -> ()
                n80 = call <vilib>:"Unset Busy.vi"("error in (no error)"=w276) -> ("error out"=w277:errorcluster)  [unwired: 1 in, 9 out]
              }
            }
          }
          event "MHM_ReadParams": Value Change {
            n81 = event-data() -> ()  [unwired: 2 out]
            n82 = flat-sequence {
              tunnel: w285 -> [w292]
              tunnel: [w290] -> w284
              tunnel: w283 -> [w289]
              tunnel: [w289] -> w282
              tunnel: [w288] -> w280
              tunnel: w279 -> [w288]
              tunnel: [w297] -> w287
              tunnel: w284 -> [w296]
              tunnel: [w294] -> w281
              tunnel: w282 -> [w294]
              tunnel: w280 -> [w293]
              tunnel: [w293] -> w278
              frame #0 {
                n83 = call <vilib>:"Set Busy.vi"("error in (no error)"=w292) -> ("error out"=w291:errorcluster)  [unwired: 3 in, 7 out]
                n84 = call "MHM Read Params.vi"("error in (no error)"=w291, "ulMHMHandle"=w289) -> ("error out"=w290:errorcluster)  [unwired: 8 in, 1 out]
              }
              frame #1 {
                n85 = local write "MHM_ReadParams"(FALSE ("MHM_ReadParams")) -> ()
                n86 = call <vilib>:"Unset Busy.vi"("error in (no error)"=w296) -> ("error out"=w297:errorcluster)  [unwired: 1 in, 9 out]
              }
            }
          }
          event "MHM_ReadStatusRegister": Value Change {
            n87 = event-data() -> ()  [unwired: 2 out]
            n88 = flat-sequence {
              tunnel: w306 -> [w312]
              tunnel: [w310] -> w304
              tunnel: w303 -> [w309]
              tunnel: [w309] -> w302
              tunnel: [w308] -> w300
              tunnel: w299 -> [w308]
              tunnel: [w317] -> w307
              tunnel: w304 -> [w316]
              tunnel: [w314] -> w301
              tunnel: w302 -> [w314]
              tunnel: w300 -> [w313]
              tunnel: [w313] -> w298
              frame #0 {
                n89 = call <vilib>:"Set Busy.vi"("error in (no error)"=w312) -> ("error out"=w311:errorcluster)  [unwired: 3 in, 7 out]
                n90 = call "MHM Read Status Register.vi"("error in (no error)"=w311, "ulMHMHandle"=w309) -> ("error out"=w310:errorcluster)  [unwired: 8 in, 1 out]
              }
              frame #1 {
                n91 = local write "MHM_ReadStatusRegister"(FALSE ("MHM_ReadStatusRegister")) -> ()
                n92 = call <vilib>:"Unset Busy.vi"("error in (no error)"=w316) -> ("error out"=w317:errorcluster)  [unwired: 1 in, 9 out]
              }
            }
          }
          event "MHM_ReadEeprom": Value Change {
            n93 = event-data() -> ()  [unwired: 2 out]
            n94 = flat-sequence {
              tunnel: w326 -> [w333]
              tunnel: [w331] -> w324
              tunnel: w323 -> [w330]
              tunnel: [w330] -> w322
              tunnel: [w329] -> w320
              tunnel: w319 -> [w329]
              tunnel: [w338] -> w327
              tunnel: w324 -> [w337]
              tunnel: [w335] -> w321
              tunnel: w322 -> [w335]
              tunnel: w320 -> [w334]
              tunnel: [w334] -> w318
              frame #0 {
                n95 = call <vilib>:"Set Busy.vi"("error in (no error)"=w333) -> ("error out"=w332:errorcluster)  [unwired: 3 in, 7 out]
                n96 = call "MHM Read Eeprom.vi"("error in (no error)"=w332, "ulEepromArea"="MHM_E2PRangeEnum", "ulMHMHandle"=w330) -> ("error out"=w331:errorcluster)  [unwired: 7 in, 1 out]
              }
              frame #1 {
                n97 = local write "MHM_ReadEeprom"(FALSE ("MHM_ReadStatusRegister")) -> ()
                n98 = call <vilib>:"Unset Busy.vi"("error in (no error)"=w337) -> ("error out"=w338:errorcluster)  [unwired: 1 in, 9 out]
              }
            }
          }
          event "MHM_GetCorrectedRegisters": Value Change {
            n99 = event-data() -> ()  [unwired: 2 out]
            n100 = flat-sequence {
              tunnel: w347 -> [w354]
              tunnel: [w352] -> w345
              tunnel: w344 -> [w351]
              tunnel: [w351] -> w343
              tunnel: [w350] -> w341
              tunnel: w340 -> [w350]
              tunnel: [w359] -> w348
              tunnel: w345 -> [w358]
              tunnel: [w356] -> w342
              tunnel: w343 -> [w356]
              tunnel: w341 -> [w355]
              tunnel: [w355] -> w339
              frame #0 {
                n101 = call <vilib>:"Set Busy.vi"("error in (no error)"=w354) -> ("error out"=w353:errorcluster)  [unwired: 3 in, 7 out]
                n102 = call "MHM Get Corrected Registers.vi"("error in (no error)"=w353, "ulMHMHandle"=w351) -> ("error out"=w352:errorcluster, "pulCorrected"=→"pulCorrected":u32[])  [unwired: 7 in, 1 out]
              }
              frame #1 {
                n103 = local write "MHM_GetCorrectedRegisters"(FALSE ("MHM_ReadStatusRegister")) -> ()
                n104 = call <vilib>:"Unset Busy.vi"("error in (no error)"=w358) -> ("error out"=w359:errorcluster)  [unwired: 1 in, 9 out]
              }
            }
          }
          event "MHM_GetParam": Value Change {
            n105 = event-data() -> ()  [unwired: 2 out]
            n106 = flat-sequence {
              tunnel: w368 -> [w376]
              tunnel: w367 -> [w371]
              tunnel: [w372] -> w366
              tunnel: [w371] -> w364
              tunnel: [w370] -> w362
              tunnel: w361 -> [w370]
              tunnel: [w381] -> w369
              tunnel: w366 -> [w380]
              tunnel: [w378] -> w363
              tunnel: w364 -> [w378]
              tunnel: w362 -> [w377]
              tunnel: [w377] -> w360
              frame #0 {
                n107 = call <vilib>:"Set Busy.vi"("error in (no error)"=w376) -> ("error out"=w375:errorcluster)  [unwired: 3 in, 7 out]
                n108 = call "MHM Get Param.vi"("error in (no error)"=w375, "ulParam"="MHM_ParamEnum", "ulMHMHandle"=w371) -> ("error out"=w372:errorcluster, "pulValue"=→"ulValue GetParam":u32)  [unwired: 6 in, 1 out]
              }
              frame #1 {
                n109 = local write "MHM_GetParam"(FALSE ("MHM_GetParam")) -> ()
                n110 = call <vilib>:"Unset Busy.vi"("error in (no error)"=w380) -> ("error out"=w381:errorcluster)  [unwired: 1 in, 9 out]
              }
            }
          }
          event "MHM_SetParam": Value Change {
            n111 = event-data() -> ()  [unwired: 2 out]
            n112 = flat-sequence {
              tunnel: w390 -> [w399]
              tunnel: w389 -> [w393]
              tunnel: [w394] -> w388
              tunnel: [w393] -> w387
              tunnel: [w392] -> w384
              tunnel: w383 -> [w392]
              tunnel: [w404] -> w391
              tunnel: w388 -> [w403]
              tunnel: [w402] -> w386
              tunnel: w387 -> [w402]
              tunnel: w384 -> [w400]
              tunnel: [w400] -> w382
              frame #0 {
                n113 = call <vilib>:"Set Busy.vi"("error in (no error)"=w399) -> ("error out"=w398:errorcluster)  [unwired: 3 in, 7 out]
                n114 = call "MHM Set Param.vi"("ulWriteVerify"="MHM_WriteVerifyEnum", "error in (no error)"=w398, "ulValue"="ulValue SetParam", "ulParam"="MHM_ParamEnum", "ulMHMHandle"=w393) -> ("error out"=w394:errorcluster)  [unwired: 5 in, 1 out]
              }
              frame #1 {
                n115 = local write "MHM_SetParam"(FALSE ("MHM_SetParam")) -> ()
                n116 = call <vilib>:"Unset Busy.vi"("error in (no error)"=w403) -> ("error out"=w404:errorcluster)  [unwired: 1 in, 9 out]
              }
            }
          }
          event "MHM_WriteParams": Value Change {
            n117 = event-data() -> ()  [unwired: 2 out]
            n118 = flat-sequence {
              tunnel: w413 -> [w421]
              tunnel: w412 -> [w417]
              tunnel: [w419] -> w411
              tunnel: [w417] -> w410
              tunnel: [w416] -> w407
              tunnel: w406 -> [w416]
              tunnel: [w426] -> w414
              tunnel: w411 -> [w425]
              tunnel: [w423] -> w409
              tunnel: w410 -> [w423]
              tunnel: w407 -> [w422]
              tunnel: [w422] -> w405
              frame #0 {
                n119 = call <vilib>:"Set Busy.vi"("error in (no error)"=w421) -> ("error out"=w420:errorcluster)  [unwired: 3 in, 7 out]
                n120 = call "MHM Write Params.vi"("error in (no error)"=w420, "ulVerify"="ulWriteVerify", "ulMHMHandle"=w417) -> ("error out"=w419:errorcluster, "pulValid"=→"pulValid":u32[])  [unwired: 6 in, 1 out]
              }
              frame #1 {
                n121 = local write "MHM_WriteParams"(FALSE ("MHM_WriteParams")) -> ()
                n122 = call <vilib>:"Unset Busy.vi"("error in (no error)"=w425) -> ("error out"=w426:errorcluster)  [unwired: 1 in, 9 out]
              }
            }
          }
          event "MHM_WriteEeprom": Value Change {
            n123 = event-data() -> ()  [unwired: 2 out]
            n124 = flat-sequence {
              tunnel: w435 -> [w438]
              tunnel: w434 -> [w441]
              tunnel: [w442] -> w433
              tunnel: [w441] -> w431
              tunnel: [w440] -> w429
              tunnel: w428 -> [w440]
              tunnel: [w443] -> w432
              tunnel: w433 -> [w444]
              tunnel: [w447] -> w430
              tunnel: w431 -> [w447]
              tunnel: w429 -> [w445]
              tunnel: [w445] -> w427
              frame #0 {
                n125 = call <vilib>:"Set Busy.vi"("error in (no error)"=w438) -> ("error out"=w437:errorcluster)  [unwired: 3 in, 7 out]
                n126 = call "MHM Write Eeprom.vi"("error in (no error)"=w437, "ulEepromArea"="MHM_E2PRangeEnum", "ulMHMHandle"=w441) -> ("error out"=w442:errorcluster)  [unwired: 7 in, 1 out]
              }
              frame #1 {
                n127 = local write "MHM_WriteEeprom"(FALSE ("MHM_WriteEeprom")) -> ()
                n128 = call <vilib>:"Unset Busy.vi"("error in (no error)"=w444) -> ("error out"=w443:errorcluster)  [unwired: 1 in, 9 out]
              }
            }
          }
          event "MHM_SetCalCfg": Value Change {
            n129 = event-data() -> ()  [unwired: 2 out]
            n130 = flat-sequence {
              tunnel: w452 -> [w463]
              tunnel: w454 -> [w460]
              tunnel: [w461] -> w457
              tunnel: [w460] -> w456
              tunnel: [w464] -> w455
              tunnel: w453 -> [w464]
              tunnel: [w465] -> w449
              tunnel: w457 -> [w466]
              tunnel: [w469] -> w450
              tunnel: w456 -> [w469]
              tunnel: w455 -> [w468]
              tunnel: [w468] -> w451
              frame #0 {
                n131 = call <vilib>:"Set Busy.vi"("error in (no error)"=w463) -> ("error out"=w462:errorcluster)  [unwired: 3 in, 7 out]
                n132 = call "MHM Set Cal Cfg.vi"("error in (no error)"=w462, "lValue"="lValue", "ulConfig"="MHM_CalCfgEnum", "ulMHMHandle"=w460) -> ("error out"=w461:errorcluster)  [unwired: 6 in, 1 out]
              }
              frame #1 {
                n133 = local write "MHM_SetCalCfg"(FALSE ("MHM_WriteEeprom")) -> ()
                n134 = call <vilib>:"Unset Busy.vi"("error in (no error)"=w466) -> ("error out"=w465:errorcluster)  [unwired: 1 in, 9 out]
              }
            }
          }
          event "MHM_GetCalCfg": Value Change {
            n135 = event-data() -> ()  [unwired: 2 out]
            n136 = flat-sequence {
              tunnel: w474 -> [w485]
              tunnel: w476 -> [w482]
              tunnel: [w483] -> w479
              tunnel: [w482] -> w478
              tunnel: [w486] -> w477
              tunnel: w475 -> [w486]
              tunnel: [w487] -> w471
              tunnel: w479 -> [w488]
              tunnel: [w491] -> w472
              tunnel: w478 -> [w491]
              tunnel: w477 -> [w490]
              tunnel: [w490] -> w473
              frame #0 {
                n137 = call <vilib>:"Set Busy.vi"("error in (no error)"=w485) -> ("error out"=w484:errorcluster)  [unwired: 3 in, 7 out]
                n138 = call "MHM Get Cal Cfg.vi"("error in (no error)"=w484, "ulConfig"="MHM_CalCfgEnum", "ulMHMHandle"=w482) -> ("error out"=w483:errorcluster, "plValue"=→"plValue":i32)  [unwired: 6 in, 1 out]
              }
              frame #1 {
                n139 = local write "MHM_GetCalCfg"(FALSE ("MHM_WriteEeprom")) -> ()
                n140 = call <vilib>:"Unset Busy.vi"("error in (no error)"=w488) -> ("error out"=w487:errorcluster)  [unwired: 1 in, 9 out]
              }
            }
          }
          event "MHM_FullAcquisition": Value Change {
            n141 = event-data() -> ()  [unwired: 2 out]
            n142 = flat-sequence {
              tunnel: w496 -> [w503]
              tunnel: w498 -> [w505]
              tunnel: [w506] -> w501
              tunnel: [w505] -> w500
              tunnel: [w507] -> w499
              tunnel: w497 -> [w507]
              tunnel: [w508] -> w493
              tunnel: w501 -> [w509]
              tunnel: [w512] -> w494
              tunnel: w500 -> [w512]
              tunnel: w499 -> [w511]
              tunnel: [w511] -> w495
              frame #0 {
                n143 = call <vilib>:"Set Busy.vi"("error in (no error)"=w503) -> ("error out"=w502:errorcluster)  [unwired: 3 in, 7 out]
                n144 = call "MHM FullAcquisition.vi"("error in (no error)"=w502, "ulCycles"="ulCycles", "ulMHMHandle"=w505) -> ("error out"=w506:errorcluster)  [unwired: 7 in, 1 out]
              }
              frame #1 {
                n145 = local write "MHM_FullAcquisition"(FALSE ("MHM_WriteEeprom")) -> ()
                n146 = call <vilib>:"Unset Busy.vi"("error in (no error)"=w509) -> ("error out"=w508:errorcluster)  [unwired: 1 in, 9 out]
              }
            }
          }
          event "MHM_FullCalibration": Value Change {
            n147 = event-data() -> ()  [unwired: 2 out]
            n148 = flat-sequence {
              tunnel: w517 -> [w524]
              tunnel: w519 -> [w527]
              tunnel: [w526] -> w522
              tunnel: [w527] -> w521
              tunnel: [w528] -> w520
              tunnel: w518 -> [w528]
              tunnel: [w529] -> w514
              tunnel: w522 -> [w530]
              tunnel: [w533] -> w515
              tunnel: w521 -> [w533]
              tunnel: w520 -> [w532]
              tunnel: [w532] -> w516
              frame #0 {
                n149 = call <vilib>:"Set Busy.vi"("error in (no error)"=w524) -> ("error out"=w523:errorcluster)  [unwired: 3 in, 7 out]
                n150 = call "MHM FullCalibration.vi"("error in (no error)"=w523, "ulCycles"="ulCycles", "ulMHMHandle"=w527) -> ("error out"=w526:errorcluster)  [unwired: 7 in, 1 out]
              }
              frame #1 {
                n151 = local write "MHM_FullCalibration"(FALSE ("MHM_WriteEeprom")) -> ()
                n152 = call <vilib>:"Unset Busy.vi"("error in (no error)"=w530) -> ("error out"=w529:errorcluster)  [unwired: 1 in, 9 out]
              }
            }
          }
          event "MHM_GetCalData": Value Change {
            n153 = event-data() -> ()  [unwired: 2 out]
            n154 = flat-sequence {
              tunnel: w538 -> [w550]
              tunnel: w540 -> [w549]
              tunnel: [w547] -> w543
              tunnel: [w549] -> w542
              tunnel: [w551] -> w541
              tunnel: w539 -> [w551]
              tunnel: [w552] -> w535
              tunnel: w543 -> [w553]
              tunnel: [w556] -> w536
              tunnel: w542 -> [w556]
              tunnel: w541 -> [w555]
              tunnel: [w555] -> w537
              frame #0 {
                n155 = call <vilib>:"Set Busy.vi"("error in (no error)"=w550) -> ("error out"=w548:errorcluster)  [unwired: 3 in, 7 out]
                n156 = call "MHM Get Cal Data.vi"("error in (no error)"=w548, "pulNumberOfBytes"="pulNumberOfBytes", "ulParam"="MHM_CalDataEnum", "ulMHMHandle"=w549) -> ("error out"=w547:errorcluster, "plData"=→"plData":i32[])  [unwired: 4 in, 2 out]
              }
              frame #1 {
                n157 = local write "MHM_GetCalData"(FALSE ("MHM_WriteEeprom")) -> ()
                n158 = call <vilib>:"Unset Busy.vi"("error in (no error)"=w553) -> ("error out"=w552:errorcluster)  [unwired: 1 in, 9 out]
              }
            }
          }
          event "MHM_SetCalData": Value Change {
            n159 = event-data() -> ()  [unwired: 2 out]
            n160 = flat-sequence {
              tunnel: w561 -> [w573]
              tunnel: w563 -> [w572]
              tunnel: [w570] -> w566
              tunnel: [w572] -> w565
              tunnel: [w574] -> w564
              tunnel: w562 -> [w574]
              tunnel: [w575] -> w558
              tunnel: w566 -> [w576]
              tunnel: [w579] -> w559
              tunnel: w565 -> [w579]
              tunnel: w564 -> [w578]
              tunnel: [w578] -> w560
              frame #0 {
                n161 = call <vilib>:"Set Busy.vi"("error in (no error)"=w573) -> ("error out"=w571:errorcluster)  [unwired: 3 in, 7 out]
                n162 = call "MHM Set Cal Data.vi"("plData"="plData", "error in (no error)"=w571, "ulNumberOfBytes"="ulNumberOfBytes", "ulParam"="MHM_CalDataEnum", "ulMHMHandle"=w572) -> ("error out"=w570:errorcluster)  [unwired: 5 in, 1 out]
              }
              frame #1 {
                n163 = local write "MHM_SetCalData"(FALSE ("MHM_WriteEeprom")) -> ()
                n164 = call <vilib>:"Unset Busy.vi"("error in (no error)"=w576) -> ("error out"=w575:errorcluster)  [unwired: 1 in, 9 out]
              }
            }
          }
          event "MHM_GetCalParam": Value Change {
            n165 = event-data() -> ()  [unwired: 2 out]
            n166 = flat-sequence {
              tunnel: w584 -> [w595]
              tunnel: w586 -> [w593]
              tunnel: [w592] -> w589
              tunnel: [w593] -> w588
              tunnel: [w596] -> w587
              tunnel: w585 -> [w596]
              tunnel: [w597] -> w581
              tunnel: w589 -> [w598]
              tunnel: [w601] -> w582
              tunnel: w588 -> [w601]
              tunnel: w587 -> [w600]
              tunnel: [w600] -> w583
              frame #0 {
                n167 = call <vilib>:"Set Busy.vi"("error in (no error)"=w595) -> ("error out"=w594:errorcluster)  [unwired: 3 in, 7 out]
                n168 = call "MHM Get Cal Param.vi"("error in (no error)"=w594, "ulParam"="MHM_CalParamEnum", "ulMHMHandle"=w593) -> ("error out"=w592:errorcluster, "plData"=→"plData":i32)  [unwired: 6 in, 1 out]
              }
              frame #1 {
                n169 = local write "MHM_GetCalParam"(FALSE ("MHM_WriteEeprom")) -> ()
                n170 = call <vilib>:"Unset Busy.vi"("error in (no error)"=w598) -> ("error out"=w597:errorcluster)  [unwired: 1 in, 9 out]
              }
            }
          }
          event "MHM_AdjustGain": Value Change {
            n171 = event-data() -> ()  [unwired: 2 out]
            n172 = flat-sequence {
              tunnel: w606 -> [w615]
              tunnel: w608 -> [w613]
              tunnel: [w612] -> w611
              tunnel: [w613] -> w610
              tunnel: [w616] -> w609
              tunnel: w607 -> [w616]
              tunnel: [w617] -> w603
              tunnel: w611 -> [w618]
              tunnel: [w621] -> w604
              tunnel: w610 -> [w621]
              tunnel: w609 -> [w620]
              tunnel: [w620] -> w605
              frame #0 {
                n173 = call <vilib>:"Set Busy.vi"("error in (no error)"=w615) -> ("error out"=w614:errorcluster)  [unwired: 3 in, 7 out]
                n174 = call "MHM Adjust Gain.vi"("error in (no error)"=w614, "ulMHMHandle"=w613) -> ("error out"=w612:errorcluster)  [unwired: 8 in, 1 out]
              }
              frame #1 {
                n175 = local write "MHM_AdjustGain"(FALSE ("MHM_WriteEeprom")) -> ()
                n176 = call <vilib>:"Unset Busy.vi"("error in (no error)"=w618) -> ("error out"=w617:errorcluster)  [unwired: 1 in, 9 out]
              }
            }
          }
          event "MHM_ActivateCalCfg": Value Change {
            n177 = event-data() -> ()  [unwired: 2 out]
            n178 = flat-sequence {
              tunnel: w626 -> [w635]
              tunnel: w628 -> [w633]
              tunnel: [w632] -> w631
              tunnel: [w633] -> w630
              tunnel: [w636] -> w629
              tunnel: w627 -> [w636]
              tunnel: [w637] -> w623
              tunnel: w631 -> [w638]
              tunnel: [w641] -> w624
              tunnel: w630 -> [w641]
              tunnel: w629 -> [w640]
              tunnel: [w640] -> w625
              frame #0 {
                n179 = call <vilib>:"Set Busy.vi"("error in (no error)"=w635) -> ("error out"=w634:errorcluster)  [unwired: 3 in, 7 out]
                n180 = call "MHM Activate Cal Cfg.vi"("error in (no error)"=w634, "ulMHMHandle"=w633) -> ("error out"=w632:errorcluster)  [unwired: 8 in, 1 out]
              }
              frame #1 {
                n181 = local write "MHM_ActivateCalCfg"(FALSE ("MHM_WriteEeprom")) -> ()
                n182 = call <vilib>:"Unset Busy.vi"("error in (no error)"=w638) -> ("error out"=w637:errorcluster)  [unwired: 1 in, 9 out]
              }
            }
          }
          event "MHM_AcquireEx": Value Change {
            n183 = event-data() -> ()  [unwired: 2 out]
            n184 = flat-sequence {
              tunnel: w646 -> [w656]
              tunnel: w648 -> [w654]
              tunnel: [w653] -> w651
              tunnel: [w654] -> w650
              tunnel: [w657] -> w649
              tunnel: w647 -> [w657]
              tunnel: [w658] -> w643
              tunnel: w651 -> [w659]
              tunnel: [w662] -> w644
              tunnel: w650 -> [w662]
              tunnel: w649 -> [w661]
              tunnel: [w661] -> w645
              frame #0 {
                n185 = call <vilib>:"Set Busy.vi"("error in (no error)"=w656) -> ("error out"=w655:errorcluster)  [unwired: 3 in, 7 out]
                n186 = call "MHM AcquireEx.vi"("error in (no error)"=w655, "ulCycles"="ulCycles", "ulMHMHandle"=w654) -> ("error out"=w653:errorcluster)  [unwired: 7 in, 1 out]
              }
              frame #1 {
                n187 = local write "MHM_AcquireEx"(FALSE ("MHM_WriteEeprom")) -> ()
                n188 = call <vilib>:"Unset Busy.vi"("error in (no error)"=w659) -> ("error out"=w658:errorcluster)  [unwired: 1 in, 9 out]
              }
            }
          }
          event "MHM_DeactivateCalCfg": Value Change {
            n189 = event-data() -> ()  [unwired: 2 out]
            n190 = flat-sequence {
              tunnel: w667 -> [w676]
              tunnel: w669 -> [w674]
              tunnel: [w673] -> w672
              tunnel: [w674] -> w671
              tunnel: [w677] -> w670
              tunnel: w668 -> [w677]
              tunnel: [w678] -> w664
              tunnel: w672 -> [w679]
              tunnel: [w682] -> w665
              tunnel: w671 -> [w682]
              tunnel: w670 -> [w681]
              tunnel: [w681] -> w666
              frame #0 {
                n191 = call <vilib>:"Set Busy.vi"("error in (no error)"=w676) -> ("error out"=w675:errorcluster)  [unwired: 3 in, 7 out]
                n192 = call "MHM Deactivate Cal Cfg.vi"("error in (no error)"=w675, "ulMHMHandle"=w674) -> ("error out"=w673:errorcluster)  [unwired: 8 in, 1 out]
              }
              frame #1 {
                n193 = local write "MHM_DeactivateCalCfg"(FALSE ("MHM_WriteEeprom")) -> ()
                n194 = call <vilib>:"Unset Busy.vi"("error in (no error)"=w679) -> ("error out"=w678:errorcluster)  [unwired: 1 in, 9 out]
              }
            }
          }
          event "MHM_AnalyzeData": Value Change {
            n195 = event-data() -> ()  [unwired: 2 out]
            n196 = flat-sequence {
              tunnel: w687 -> [w696]
              tunnel: w689 -> [w694]
              tunnel: [w693] -> w692
              tunnel: [w694] -> w691
              tunnel: [w697] -> w690
              tunnel: w688 -> [w697]
              tunnel: [w698] -> w684
              tunnel: w692 -> [w699]
              tunnel: [w702] -> w685
              tunnel: w691 -> [w702]
              tunnel: w690 -> [w701]
              tunnel: [w701] -> w686
              frame #0 {
                n197 = call <vilib>:"Set Busy.vi"("error in (no error)"=w696) -> ("error out"=w695:errorcluster)  [unwired: 3 in, 7 out]
                n198 = call "MHM Analyze Data.vi"("error in (no error)"=w695, "ulMHMHandle"=w694) -> ("error out"=w693:errorcluster)  [unwired: 8 in, 1 out]
              }
              frame #1 {
                n199 = local write "MHM_AnalyzeData"(FALSE ("MHM_WriteEeprom")) -> ()
                n200 = call <vilib>:"Unset Busy.vi"("error in (no error)"=w699) -> ("error out"=w698:errorcluster)  [unwired: 1 in, 9 out]
              }
            }
          }
          event "MHM_Adjust": Value Change {
            n201 = event-data() -> ()  [unwired: 2 out]
            n202 = flat-sequence {
              tunnel: w707 -> [w717]
              tunnel: w709 -> [w715]
              tunnel: [w714] -> w712
              tunnel: [w715] -> w711
              tunnel: [w718] -> w710
              tunnel: w708 -> [w718]
              tunnel: [w719] -> w704
              tunnel: w712 -> [w720]
              tunnel: [w723] -> w705
              tunnel: w711 -> [w723]
              tunnel: w710 -> [w722]
              tunnel: [w722] -> w706
              frame #0 {
                n203 = call <vilib>:"Set Busy.vi"("error in (no error)"=w717) -> ("error out"=w716:errorcluster)  [unwired: 3 in, 7 out]
                n204 = call "MHM Adjust.vi"("error in (no error)"=w716, "ulWriteVerify"="MHM_WriteVerifyEnum", "ulMHMHandle"=w715) -> ("error out"=w714:errorcluster)  [unwired: 7 in, 1 out]
              }
              frame #1 {
                n205 = local write "MHM_Adjust"(FALSE ("MHM_WriteEeprom")) -> ()
                n206 = call <vilib>:"Unset Busy.vi"("error in (no error)"=w720) -> ("error out"=w719:errorcluster)  [unwired: 1 in, 9 out]
              }
            }
          }
          event "MHM_ReadEdsParams": Value Change {
            n207 = event-data() -> ()  [unwired: 2 out]
            n208 = flat-sequence {
              tunnel: w732 -> [w735]
              tunnel: w731 -> [w738]
              tunnel: [w738] -> w730
              tunnel: [w737] -> w728
              tunnel: w727 -> [w737]
              tunnel: [w736] -> w725
              tunnel: [w743] -> w729
              tunnel: w730 -> [w743]
              tunnel: w728 -> [w742]
              tunnel: [w742] -> w726
              tunnel: [w739] -> w724
              tunnel: w725 -> [w740]
              frame #0 {
                n209 = call <vilib>:"Set Busy.vi"("error in (no error)"=w735) -> ("error out"=w734:errorcluster)  [unwired: 3 in, 7 out]
                n210 = call "MHM Read Eds Params.vi"("error in (no error)"=w734, "ulMHMHandle"=w738) -> ("error out"=w736:errorcluster)  [unwired: 8 in, 1 out]
              }
              frame #1 {
                n211 = local write "MHM_ReadEdsParams"(FALSE ("MHM_ReadEdsParams")) -> ()
                n212 = call <vilib>:"Unset Busy.vi"("error in (no error)"=w740) -> ("error out"=w739:errorcluster)  [unwired: 1 in, 9 out]
              }
            }
          }
          event "MHM_SetEdsParam": Value Change {
            n213 = event-data() -> ()  [unwired: 2 out]
            n214 = flat-sequence {
              tunnel: w752 -> [w755]
              tunnel: w751 -> [w757]
              tunnel: [w758] -> w750
              tunnel: [w757] -> w748
              tunnel: [w756] -> w746
              tunnel: w745 -> [w756]
              tunnel: w750 -> [w762]
              tunnel: [w761] -> w749
              tunnel: [w765] -> w747
              tunnel: w748 -> [w765]
              tunnel: w746 -> [w764]
              tunnel: [w764] -> w744
              frame #0 {
                n215 = call <vilib>:"Set Busy.vi"("error in (no error)"=w755) -> ("error out"=w754:errorcluster)  [unwired: 3 in, 7 out]
                n216 = call "MHM Set Eds Param.vi"("error in (no error)"=w754, "ulValue"="ulValue", "ulParam"="MHM_EdsParamEnum", "ulMHMHandle"=w757) -> ("error out"=w758:errorcluster)  [unwired: 6 in, 1 out]
              }
              frame #1 {
                n217 = local write "MHM_SetEdsParam"(FALSE ("MHM_SetEdsParam")) -> ()
                n218 = call <vilib>:"Unset Busy.vi"("error in (no error)"=w762) -> ("error out"=w761:errorcluster)  [unwired: 1 in, 9 out]
              }
            }
          }
          event "MHM_UpdateEds": Value Change {
            n219 = event-data() -> ()  [unwired: 2 out]
            n220 = flat-sequence {
              tunnel: w774 -> [w777]
              tunnel: w773 -> [w779]
              tunnel: [w780] -> w772
              tunnel: [w779] -> w770
              tunnel: [w778] -> w768
              tunnel: w767 -> [w778]
              tunnel: w772 -> [w782]
              tunnel: [w781] -> w771
              tunnel: [w785] -> w769
              tunnel: w770 -> [w785]
              tunnel: w768 -> [w784]
              tunnel: [w784] -> w766
              frame #0 {
                n221 = call <vilib>:"Set Busy.vi"("error in (no error)"=w777) -> ("error out"=w776:errorcluster)  [unwired: 3 in, 7 out]
                n222 = call "MHM Update EDS.vi"("error in (no error)"=w776, "ulMHMHandle"=w779) -> ("error out"=w780:errorcluster)  [unwired: 8 in, 1 out]
              }
              frame #1 {
                n223 = local write "MHM_UpdateEds"(FALSE ("MHM_SetEdsParam")) -> ()
                n224 = call <vilib>:"Unset Busy.vi"("error in (no error)"=w782) -> ("error out"=w781:errorcluster)  [unwired: 1 in, 9 out]
              }
            }
          }
          event "MHM_GetEdsParam": Value Change {
            n225 = event-data() -> ()  [unwired: 2 out]
            n226 = flat-sequence {
              tunnel: w794 -> [w797]
              tunnel: w793 -> [w801]
              tunnel: [w801] -> w792
              tunnel: [w800] -> w790
              tunnel: w789 -> [w800]
              tunnel: [w798] -> w787
              tunnel: [w807] -> w791
              tunnel: w792 -> [w807]
              tunnel: w790 -> [w806]
              tunnel: [w806] -> w788
              tunnel: [w803] -> w786
              tunnel: w787 -> [w804]
              frame #0 {
                n227 = call <vilib>:"Set Busy.vi"("error in (no error)"=w797) -> ("error out"=w796:errorcluster)  [unwired: 3 in, 7 out]
                n228 = call "MHM Get Eds Param.vi"("error in (no error)"=w796, "ulParam"="EdsParamEnum", "ulMHMHandle"=w801) -> ("error out"=w798:errorcluster, "pulValue"=→"pulValue 2":u32)  [unwired: 6 in, 1 out]
              }
              frame #1 {
                n229 = local write "MHM_GetEdsParam"(FALSE ("MHM_GetEdsParam")) -> ()
                n230 = call <vilib>:"Unset Busy.vi"("error in (no error)"=w804) -> ("error out"=w803:errorcluster)  [unwired: 1 in, 9 out]
              }
            }
          }
          event "MHM_WriteCommand": Value Change {
            n231 = event-data() -> ()  [unwired: 2 out]
            n232 = flat-sequence {
              tunnel: w815 -> [w823]
              tunnel: [w821] -> w814
              tunnel: w813 -> [w820]
              tunnel: [w820] -> w812
              tunnel: [w819] -> w810
              tunnel: w809 -> [w819]
              tunnel: [w828] -> w817
              tunnel: w814 -> [w827]
              tunnel: [w826] -> w811
              tunnel: w812 -> [w826]
              tunnel: w810 -> [w824]
              tunnel: [w824] -> w808
              frame #0 {
                n233 = call <vilib>:"Set Busy.vi"("error in (no error)"=w823) -> ("error out"=w822:errorcluster)  [unwired: 3 in, 7 out]
                n234 = call "MHM Write Command.vi"("error in (no error)"=w822, "ulCommand"="ulCommand", "ulMHMHandle"=w820) -> ("error out"=w821:errorcluster)  [unwired: 7 in, 1 out]
              }
              frame #1 {
                n235 = local write "MHM_WriteCommand"(FALSE ("MHM_WriteCommand")) -> ()
                n236 = call <vilib>:"Unset Busy.vi"("error in (no error)"=w827) -> ("error out"=w828:errorcluster)  [unwired: 1 in, 9 out]
              }
            }
          }
          event "MHM_Preset": Value Change {
            n237 = event-data() -> ()  [unwired: 2 out]
            n238 = flat-sequence {
              tunnel: w836 -> [w843]
              tunnel: [w841] -> w835
              tunnel: w834 -> [w840]
              tunnel: [w840] -> w833
              tunnel: [w839] -> w831
              tunnel: w830 -> [w839]
              tunnel: [w848] -> w838
              tunnel: w835 -> [w847]
              tunnel: [w846] -> w832
              tunnel: w833 -> [w846]
              tunnel: w831 -> [w844]
              tunnel: [w844] -> w829
              frame #0 {
                n239 = call <vilib>:"Set Busy.vi"("error in (no error)"=w843) -> ("error out"=w842:errorcluster)  [unwired: 3 in, 7 out]
                n240 = call "MHM Preset.vi"("error in (no error)"=w842, "ulMHMHandle"=w840) -> ("error out"=w841:errorcluster)  [unwired: 8 in, 1 out]
              }
              frame #1 {
                n241 = local write "MHM_Preset"(FALSE ("MHM_WriteCommand")) -> ()
                n242 = call <vilib>:"Unset Busy.vi"("error in (no error)"=w847) -> ("error out"=w848:errorcluster)  [unwired: 1 in, 9 out]
              }
            }
          }
          event "MHM_WritePorts": Value Change {
            n243 = event-data() -> ()  [unwired: 2 out]
            n244 = flat-sequence {
              tunnel: w858 -> [w864]
              tunnel: [w862] -> w857
              tunnel: w854 -> [w860]
              tunnel: [w860] -> w853
              tunnel: [w859] -> w851
              tunnel: w850 -> [w859]
              tunnel: [w869] -> w856
              tunnel: w857 -> [w868]
              tunnel: [w867] -> w852
              tunnel: w853 -> [w867]
              tunnel: w851 -> [w865]
              tunnel: [w865] -> w849
              frame #0 {
                n245 = call <vilib>:"Set Busy.vi"("error in (no error)"=w864) -> ("error out"=w863:errorcluster)  [unwired: 3 in, 7 out]
                n246 = call "MHM Write Ports.vi"("error in (no error)"=w863, "ulPorts"="ulPorts", "ulMHMHandle"=w860) -> ("error out"=w862:errorcluster)  [unwired: 7 in, 1 out]
              }
              frame #1 {
                n247 = local write "MHM_WritePorts"(FALSE ("MHM_WritePorts")) -> ()
                n248 = call <vilib>:"Unset Busy.vi"("error in (no error)"=w868) -> ("error out"=w869:errorcluster)  [unwired: 1 in, 9 out]
              }
            }
          }
          event "MHM_ReadPorts": Value Change {
            n249 = event-data() -> ()  [unwired: 2 out]
            n250 = flat-sequence {
              tunnel: w878 -> [w885]
              tunnel: [w883] -> w877
              tunnel: w876 -> [w882]
              tunnel: [w882] -> w875
              tunnel: [w880] -> w872
              tunnel: w871 -> [w880]
              tunnel: [w890] -> w879
              tunnel: w877 -> [w889]
              tunnel: [w888] -> w874
              tunnel: w875 -> [w888]
              tunnel: w872 -> [w886]
              tunnel: [w886] -> w870
              frame #0 {
                n251 = call <vilib>:"Set Busy.vi"("error in (no error)"=w885) -> ("error out"=w884:errorcluster)  [unwired: 3 in, 7 out]
                n252 = call "MHM Read Ports.vi"("error in (no error)"=w884, "ulMHMHandle"=w882) -> ("error out"=w883:errorcluster, "pulPorts"=→"pulPorts":u32)  [unwired: 7 in, 1 out]
              }
              frame #1 {
                n253 = local write "MHM_ReadPorts"(FALSE ("MHM_ReadPorts")) -> ()
                n254 = call <vilib>:"Unset Busy.vi"("error in (no error)"=w889) -> ("error out"=w890:errorcluster)  [unwired: 1 in, 9 out]
              }
            }
          }
          event "MHM_LoadParams": Value Change {
            n255 = event-data() -> ()  [unwired: 2 out]
            n256 = flat-sequence {
              tunnel: w900 -> [w906]
              tunnel: [w904] -> w899
              tunnel: w898 -> [w902]
              tunnel: [w902] -> w897
              tunnel: [w901] -> w893
              tunnel: w892 -> [w901]
              tunnel: [w911] -> w894
              tunnel: w899 -> [w910]
              tunnel: [w909] -> w896
              tunnel: w897 -> [w909]
              tunnel: w893 -> [w907]
              tunnel: [w907] -> w891
              frame #0 {
                n257 = call <vilib>:"Set Busy.vi"("error in (no error)"=w906) -> ("error out"=w905:errorcluster)  [unwired: 3 in, 7 out]
                n258 = call "MHM Load Params.vi"("error in (no error)"=w905, "pcFilename"="pcFilename", "ulMHMHandle"=w902) -> ("error out"=w904:errorcluster)  [unwired: 7 in, 1 out]
              }
              frame #1 {
                n259 = local write "MHM_LoadParams"(FALSE ("MHM_LoadParams")) -> ()
                n260 = call <vilib>:"Unset Busy.vi"("error in (no error)"=w910) -> ("error out"=w911:errorcluster)  [unwired: 1 in, 9 out]
              }
            }
          }
          event "MHM_SaveParams": Value Change {
            n261 = event-data() -> ()  [unwired: 2 out]
            n262 = flat-sequence {
              tunnel: w920 -> [w927]
              tunnel: [w925] -> w919
              tunnel: w918 -> [w923]
              tunnel: [w923] -> w917
              tunnel: [w922] -> w914
              tunnel: w913 -> [w922]
              tunnel: [w932] -> w921
              tunnel: w919 -> [w931]
              tunnel: [w930] -> w916
              tunnel: w917 -> [w930]
              tunnel: w914 -> [w928]
              tunnel: [w928] -> w912
              frame #0 {
                n263 = call <vilib>:"Set Busy.vi"("error in (no error)"=w927) -> ("error out"=w926:errorcluster)  [unwired: 3 in, 7 out]
                n264 = call "MHM Save Params.vi"("error in (no error)"=w926, "pcFilename"="pcFilename", "ulMHMHandle"=w923) -> ("error out"=w925:errorcluster)  [unwired: 7 in, 1 out]
              }
              frame #1 {
                n265 = local write "MHM_SaveParams"(FALSE ("MHM_SaveParams")) -> ()
                n266 = call <vilib>:"Unset Busy.vi"("error in (no error)"=w931) -> ("error out"=w932:errorcluster)  [unwired: 1 in, 9 out]
              }
            }
          }
          event "MHM_GetDLLVersion": Value Change {
            n267 = event-data() -> ()  [unwired: 2 out]
            n268 = flat-sequence {
              tunnel: w941 -> [w948]
              tunnel: [w946] -> w940
              tunnel: [w944] -> w938
              tunnel: w937 -> [w944]
              tunnel: [w943] -> w935
              tunnel: w934 -> [w943]
              tunnel: [w953] -> w942
              tunnel: w940 -> [w952]
              tunnel: w938 -> [w950]
              tunnel: [w950] -> w936
              tunnel: w935 -> [w949]
              tunnel: [w949] -> w933
              frame #0 {
                n269 = call <vilib>:"Set Busy.vi"("error in (no error)"=w948) -> ("error out"=w947:errorcluster)  [unwired: 3 in, 7 out]
                n270 = call "MHM Get DLL Version.vi"("error in (no error)"=w947) -> ("error out"=w946:errorcluster, "pulDllVersion"=→"pulDllVersion":u32[])  [unwired: 8 in, 1 out]
              }
              frame #1 {
                n271 = local write "MHM_GetDLLVersion"(FALSE ("MHM_GetDLLVersion")) -> ()
                n272 = call <vilib>:"Unset Busy.vi"("error in (no error)"=w952) -> ("error out"=w953:errorcluster)  [unwired: 1 in, 9 out]
              }
            }
          }
          event "MHM_SPIActivate": Value Change {
            n273 = event-data() -> ()  [unwired: 2 out]
            n274 = flat-sequence {
              tunnel: w962 -> [w969]
              tunnel: [w967] -> w960
              tunnel: w959 -> [w966]
              tunnel: [w966] -> w958
              tunnel: [w964] -> w956
              tunnel: w955 -> [w964]
              tunnel: [w974] -> w963
              tunnel: w960 -> [w973]
              tunnel: [w972] -> w957
              tunnel: w958 -> [w972]
              tunnel: w956 -> [w970]
              tunnel: [w970] -> w954
              frame #0 {
                n275 = call <vilib>:"Set Busy.vi"("error in (no error)"=w969) -> ("error out"=w968:errorcluster)  [unwired: 3 in, 7 out]
                n276 = call "MHM Spi Activate.vi"("error in (no error)"=w968, "ulData"="ulData", "ulMHMHandle"=w966) -> ("error out"=w967:errorcluster)  [unwired: 7 in, 1 out]
              }
              frame #1 {
                n277 = local write "MHM_SPIActivate"(FALSE ("MHM_SPIActivate")) -> ()
                n278 = call <vilib>:"Unset Busy.vi"("error in (no error)"=w973) -> ("error out"=w974:errorcluster)  [unwired: 1 in, 9 out]
              }
            }
          }
          event "MHM_GetLastError": Value Change {
            n279 = event-data() -> ()  [unwired: 2 out]
            n280 = flat-sequence {
              tunnel: w983 -> [w992]
              tunnel: [w990] -> w981
              tunnel: w980 -> [w989]
              tunnel: [w989] -> w979
              tunnel: [w988] -> w977
              tunnel: w976 -> [w988]
              tunnel: [w997] -> w984
              tunnel: w981 -> [w996]
              tunnel: [w995] -> w978
              tunnel: w979 -> [w995]
              tunnel: w977 -> [w993]
              tunnel: [w993] -> w975
              frame #0 {
                n281 = call <vilib>:"Set Busy.vi"("error in (no error)"=w992) -> ("error out"=w991:errorcluster)  [unwired: 3 in, 7 out]
                n282 = call "MHM Get Last Error.vi"("error in (no error)"=w991, "ulMHMHandle"=w989) -> ("error out"=w990:errorcluster, "pulErrorType"=→"MHM_ErrorTypeEnum":u32, "pulLastError"=→"pulLastError":u32, "pcErrorText"=→"pcErrorText":string)  [unwired: 5 in, 1 out]
              }
              frame #1 {
                n283 = local write "MHM_GetLastError"(FALSE ("MHM_SPIActivate")) -> ()
                n284 = call <vilib>:"Unset Busy.vi"("error in (no error)"=w996) -> ("error out"=w997:errorcluster)  [unwired: 1 in, 9 out]
              }
            }
          }
          event "MHM_SetRegister": Value Change {
            n285 = event-data() -> ()  [unwired: 2 out]
            n286 = flat-sequence {
              tunnel: w1006 -> [w1015]
              tunnel: [w1013] -> w1005
              tunnel: w1004 -> [w1010]
              tunnel: [w1010] -> w1003
              tunnel: [w1008] -> w1000
              tunnel: w999 -> [w1008]
              tunnel: [w1020] -> w1007
              tunnel: w1005 -> [w1019]
              tunnel: w1003 -> [w1018]
              tunnel: [w1018] -> w1002
              tunnel: w1000 -> [w1016]
              tunnel: [w1016] -> w998
              frame #0 {
                n287 = call <vilib>:"Set Busy.vi"("error in (no error)"=w1015) -> ("error out"=w1014:errorcluster)  [unwired: 3 in, 7 out]
                n288 = call "MHM Set Register.vi"("ulWriteVerify"="MHM_WriteVerifyEnum 2", "error in (no error)"=w1014, "ulValue"="ulValue 2", "ulAdr"="ulAdr", "ulMHMHandle"=w1010) -> ("error out"=w1013:errorcluster)  [unwired: 5 in, 1 out]
              }
              frame #1 {
                n289 = local write "MHM_SetRegister"(FALSE ("MHM_SetRegister")) -> ()
                n290 = call <vilib>:"Unset Busy.vi"("error in (no error)"=w1019) -> ("error out"=w1020:errorcluster)  [unwired: 1 in, 9 out]
              }
            }
          }
          event "MHM_GetRegister": Value Change {
            n291 = event-data() -> ()  [unwired: 2 out]
            n292 = flat-sequence {
              tunnel: w1028 -> [w1037]
              tunnel: w1027 -> [w1035]
              tunnel: [w1035] -> w1026
              tunnel: [w1034] -> w1024
              tunnel: [w1031] -> w1023
              tunnel: w1022 -> [w1031]
              tunnel: [w1042] -> w1030
              tunnel: [w1041] -> w1025
              tunnel: w1026 -> [w1041]
              tunnel: w1024 -> [w1040]
              tunnel: w1023 -> [w1038]
              tunnel: [w1038] -> w1021
              frame #0 {
                n293 = call <vilib>:"Set Busy.vi"("error in (no error)"=w1037) -> ("error out"=w1036:errorcluster)  [unwired: 3 in, 7 out]
                n294 = call "MHM Get Register.vi"("error in (no error)"=w1036, "ulAdr"="ulAdr", "ulMHMHandle"=w1035) -> ("error out"=w1034:errorcluster, "pulValue"=→"pulValue":u32)  [unwired: 6 in, 1 out]
              }
              frame #1 {
                n295 = local write "MHM_GetRegister"(FALSE ("MHM_GetRegister")) -> ()
                n296 = call <vilib>:"Unset Busy.vi"("error in (no error)"=w1040) -> ("error out"=w1042:errorcluster)  [unwired: 1 in, 9 out]
              }
            }
          }
          event "MHM_WriteRegister": Value Change {
            n297 = event-data() -> ()  [unwired: 2 out]
            n298 = flat-sequence {
              tunnel: w1051 -> [w1060]
              tunnel: [w1058] -> w1049
              tunnel: w1048 -> [w1054]
              tunnel: [w1054] -> w1047
              tunnel: [w1053] -> w1045
              tunnel: w1044 -> [w1053]
              tunnel: [w1065] -> w1052
              tunnel: w1049 -> [w1064]
              tunnel: [w1062] -> w1046
              tunnel: w1047 -> [w1062]
              tunnel: w1045 -> [w1061]
              tunnel: [w1061] -> w1043
              frame #0 {
                n299 = call <vilib>:"Set Busy.vi"("error in (no error)"=w1060) -> ("error out"=w1059:errorcluster)  [unwired: 3 in, 7 out]
                n300 = call "MHM Write Register.vi"("pulData"="pulData", "error in (no error)"=w1059, "pulNumberOfBytes"="pulNumberOfBytes", "ulAdr"="ulAdr 3", "ulMHMHandle"=w1054) -> ("error out"=w1058:errorcluster)  [unwired: 4 in, 2 out]
              }
              frame #1 {
                n301 = local write "MHM_WriteRegister"(FALSE ("MHM_WriteRegister")) -> ()
                n302 = call <vilib>:"Unset Busy.vi"("error in (no error)"=w1064) -> ("error out"=w1065:errorcluster)  [unwired: 1 in, 9 out]
              }
            }
          }
          event "MHM_ReadRegister": Value Change {
            n303 = event-data() -> ()  [unwired: 2 out]
            n304 = flat-sequence {
              tunnel: w1073 -> [w1083]
              tunnel: [w1081] -> w1072
              tunnel: w1071 -> [w1080]
              tunnel: [w1080] -> w1070
              tunnel: [w1076] -> w1068
              tunnel: w1067 -> [w1076]
              tunnel: [w1088] -> w1075
              tunnel: w1072 -> [w1087]
              tunnel: [w1085] -> w1069
              tunnel: w1070 -> [w1085]
              tunnel: w1068 -> [w1084]
              tunnel: [w1084] -> w1066
              frame #0 {
                n305 = call <vilib>:"Set Busy.vi"("error in (no error)"=w1083) -> ("error out"=w1082:errorcluster)  [unwired: 3 in, 7 out]
                n306 = call "MHM Read Register.vi"("error in (no error)"=w1082, "pulNumberOfBytes"="pulNumberOfBytes", "ulAdr"="ulAdr", "ulMHMHandle"=w1080) -> ("error out"=w1081:errorcluster, "pulData"=→"pulData":u32[])  [unwired: 4 in, 2 out]
              }
              frame #1 {
                n307 = local write "MHM_ReadRegister"(FALSE ("MHM_ReadRegister")) -> ()
                n308 = call <vilib>:"Unset Busy.vi"("error in (no error)"=w1087) -> ("error out"=w1088:errorcluster)  [unwired: 1 in, 9 out]
              }
            }
          }
          event "MHM_SaveRegister": Value Change {
            n309 = event-data() -> ()  [unwired: 2 out]
            n310 = flat-sequence {
              tunnel: w1097 -> [w1107]
              tunnel: [w1105] -> w1096
              tunnel: w1095 -> [w1104]
              tunnel: [w1104] -> w1094
              tunnel: [w1099] -> w1091
              tunnel: w1090 -> [w1099]
              tunnel: [w1112] -> w1098
              tunnel: w1096 -> [w1111]
              tunnel: [w1110] -> w1093
              tunnel: w1094 -> [w1110]
              tunnel: w1091 -> [w1108]
              tunnel: [w1108] -> w1089
              frame #0 {
                n311 = call <vilib>:"Set Busy.vi"("error in (no error)"=w1107) -> ("error out"=w1106:errorcluster)  [unwired: 3 in, 7 out]
                n312 = call "MHM Save Register.vi"("pulData"="pulData 3", "pulNumerOfBytes"="pulNumberOfBytes5", "error in (no error)"=w1106, "ulAdr"="ulAdr 5", "pcFilename"="pcFilename 3", "ulMHMHandle"=w1104) -> ("error out"=w1105:errorcluster)  [unwired: 4 in, 1 out]
              }
              frame #1 {
                n313 = local write "MHM_SaveRegister"(FALSE ("MHM_SaveRegister")) -> ()
                n314 = call <vilib>:"Unset Busy.vi"("error in (no error)"=w1111) -> ("error out"=w1112:errorcluster)  [unwired: 1 in, 9 out]
              }
            }
          }
          event "MHM_LoadRegister": Value Change {
            n315 = event-data() -> ()  [unwired: 2 out]
            n316 = flat-sequence {
              tunnel: w1121 -> [w1131]
              tunnel: [w1129] -> w1120
              tunnel: w1119 -> [w1128]
              tunnel: [w1128] -> w1118
              tunnel: [w1123] -> w1115
              tunnel: w1114 -> [w1123]
              tunnel: [w1136] -> w1122
              tunnel: w1120 -> [w1135]
              tunnel: [w1133] -> w1117
              tunnel: w1118 -> [w1133]
              tunnel: w1115 -> [w1132]
              tunnel: [w1132] -> w1113
              frame #0 {
                n317 = call <vilib>:"Set Busy.vi"("error in (no error)"=w1131) -> ("error out"=w1130:errorcluster)  [unwired: 3 in, 7 out]
                n318 = call "MHM Load Register.vi"("pulNumerOfBytes"="pulNumerOfBytes", "error in (no error)"=w1130, "ulAdr"="ulAdr", "pcFilename"="pcFilename", "ulMHMHandle"=w1128) -> ("error out"=w1129:errorcluster, "pulData"=→"pulData":u32[])  [unwired: 3 in, 2 out]
              }
              frame #1 {
                n319 = local write "MHM_LoadRegister"(FALSE ("MHM_LoadRegister")) -> ()
                n320 = call <vilib>:"Unset Busy.vi"("error in (no error)"=w1135) -> ("error out"=w1136:errorcluster)  [unwired: 1 in, 9 out]
              }
            }
          }
          event "MHM_WriteRegister_I2C": Value Change {
            n321 = event-data() -> ()  [unwired: 2 out]
            n322 = flat-sequence {
              tunnel: w1145 -> [w1155]
              tunnel: [w1153] -> w1144
              tunnel: w1143 -> [w1152]
              tunnel: [w1152] -> w1142
              tunnel: [w1151] -> w1139
              tunnel: w1138 -> [w1151]
              tunnel: [w1160] -> w1146
              tunnel: w1144 -> [w1159]
              tunnel: [w1157] -> w1141
              tunnel: w1142 -> [w1157]
              tunnel: w1139 -> [w1156]
              tunnel: [w1156] -> w1137
              frame #0 {
                n323 = call <vilib>:"Set Busy.vi"("error in (no error)"=w1155) -> ("error out"=w1154:errorcluster)  [unwired: 3 in, 7 out]
                n324 = call "MHM Write Register I2C.vi"("pulData"="pulData", "ulI2CSlaveAdr"="ulI2CSlaveAdr", "error in (no error)"=w1154, "ulNumberOfBytes"="ulNumberOfBytes", "ulAdr"="ulAdr", "ulMHMHandle"=w1152) -> ("error out (no error)"=w1153:errorcluster)  [unwired: 4 in, 1 out]
              }
              frame #1 {
                n325 = local write "MHM_WriteRegister_I2C"(FALSE ("MHM_LoadRegister")) -> ()
                n326 = call <vilib>:"Unset Busy.vi"("error in (no error)"=w1159) -> ("error out"=w1160:errorcluster)  [unwired: 1 in, 9 out]
              }
            }
          }
          event "MHM_ReadRegister_I2C": Value Change {
            n327 = event-data() -> ()  [unwired: 2 out]
            n328 = flat-sequence {
              tunnel: w1169 -> [w1179]
              tunnel: [w1177] -> w1168
              tunnel: w1167 -> [w1176]
              tunnel: [w1176] -> w1166
              tunnel: [w1175] -> w1163
              tunnel: w1162 -> [w1175]
              tunnel: [w1184] -> w1170
              tunnel: w1168 -> [w1183]
              tunnel: [w1181] -> w1165
              tunnel: w1166 -> [w1181]
              tunnel: w1163 -> [w1180]
              tunnel: [w1180] -> w1161
              frame #0 {
                n329 = call <vilib>:"Set Busy.vi"("error in (no error)"=w1179) -> ("error out"=w1178:errorcluster)  [unwired: 3 in, 7 out]
                n330 = call "MHM Read Register I2C.vi"("ulI2CSlaveAdr"="ulI2CSlaveAdr", "error in (no error)"=w1178, "ulNumberOfBytes"="pulNumberOfBytes", "ulAdr"="ulAdr", "ulMHMHandle"=w1176) -> ("error out (no error)"=w1177:errorcluster, "pulData"=→"pulData":u32[])  [unwired: 4 in, 1 out]
              }
              frame #1 {
                n331 = local write "MHM_ReadRegister_I2C"(FALSE ("MHM_LoadRegister")) -> ()
                n332 = call <vilib>:"Unset Busy.vi"("error in (no error)"=w1183) -> ("error out"=w1184:errorcluster)  [unwired: 1 in, 9 out]
              }
            }
          }
          event "MHM_WriteRegister_I2C_EX": Value Change {
            n333 = event-data() -> ()  [unwired: 2 out]
            n334 = flat-sequence {
              tunnel: w1193 -> [w1203]
              tunnel: [w1201] -> w1192
              tunnel: w1191 -> [w1200]
              tunnel: [w1200] -> w1190
              tunnel: [w1199] -> w1187
              tunnel: w1186 -> [w1199]
              tunnel: [w1208] -> w1194
              tunnel: w1192 -> [w1207]
              tunnel: [w1205] -> w1189
              tunnel: w1190 -> [w1205]
              tunnel: w1187 -> [w1204]
              tunnel: [w1204] -> w1185
              frame #0 {
                n335 = call <vilib>:"Set Busy.vi"("error in (no error)"=w1203) -> ("error out"=w1202:errorcluster)  [unwired: 3 in, 7 out]
                n336 = call "MHM Write Register I2C Ex.vi"("pulValid"="pulValid", "pulData"="pulData", "error in (no error)"=w1202, "ulI2CSlaveAdr"="ulI2CSlaveAdr", "ulArraySize"="ulArraySize", "ulMHMHandle"=w1200) -> ("error out (no error)"=w1201:errorcluster)  [unwired: 4 in, 1 out]
              }
              frame #1 {
                n337 = local write "MHM_WriteRegister_I2C_EX"(FALSE ("MHM_LoadRegister")) -> ()
                n338 = call <vilib>:"Unset Busy.vi"("error in (no error)"=w1207) -> ("error out"=w1208:errorcluster)  [unwired: 1 in, 9 out]
              }
            }
          }
          event "MHM_LoadRegister_EX": Value Change {
            n339 = event-data() -> ()  [unwired: 2 out]
            n340 = flat-sequence {
              tunnel: w1217 -> [w1227]
              tunnel: [w1225] -> w1216
              tunnel: w1215 -> [w1224]
              tunnel: [w1224] -> w1214
              tunnel: [w1223] -> w1211
              tunnel: w1210 -> [w1223]
              tunnel: [w1232] -> w1218
              tunnel: w1216 -> [w1231]
              tunnel: [w1229] -> w1213
              tunnel: w1214 -> [w1229]
              tunnel: w1211 -> [w1228]
              tunnel: [w1228] -> w1209
              frame #0 {
                n341 = call <vilib>:"Set Busy.vi"("error in (no error)"=w1227) -> ("error out"=w1226:errorcluster)  [unwired: 3 in, 7 out]
                n342 = call "MHM Load Register Ex.vi"("error in (no error)"=w1226, "ulArraySize"="ulArraySize", "pcFilename"="pcFilename", "ulMHMHandle"=w1224) -> ("error out (no error)"=w1225:errorcluster, "pulValid"=→"pulValid":u32[], "pulData"=→"pulData":u32[])  [unwired: 4 in, 1 out]
              }
              frame #1 {
                n343 = local write "MHM_LoadRegister_EX"(FALSE ("MHM_LoadRegister")) -> ()
                n344 = call <vilib>:"Unset Busy.vi"("error in (no error)"=w1231) -> ("error out"=w1232:errorcluster)  [unwired: 1 in, 9 out]
              }
            }
          }
          event "MHM_SaveRegister_EX": Value Change {
            n345 = event-data() -> ()  [unwired: 2 out]
            n346 = flat-sequence {
              tunnel: w1241 -> [w1251]
              tunnel: [w1249] -> w1240
              tunnel: w1239 -> [w1248]
              tunnel: [w1248] -> w1238
              tunnel: [w1247] -> w1235
              tunnel: w1234 -> [w1247]
              tunnel: [w1256] -> w1242
              tunnel: w1240 -> [w1255]
              tunnel: [w1253] -> w1237
              tunnel: w1238 -> [w1253]
              tunnel: w1235 -> [w1252]
              tunnel: [w1252] -> w1233
              frame #0 {
                n347 = call <vilib>:"Set Busy.vi"("error in (no error)"=w1251) -> ("error out"=w1250:errorcluster)  [unwired: 3 in, 7 out]
                n348 = call "MHM Save Register Ex.vi"("pulData"="pulData", "pulNumberOfBytes"="pulNumberOfBytes", "error in (no error)"=w1250, "ulAdr"="ulAdr", "pcFilename"="pcFilename", "ulMHMHandle"=w1248) -> ("error out (no error)"=w1249:errorcluster)  [unwired: 3 in, 2 out]
              }
              frame #1 {
                n349 = local write "MHM_SaveRegister_EX"(FALSE ("MHM_LoadRegister")) -> ()
                n350 = call <vilib>:"Unset Busy.vi"("error in (no error)"=w1255) -> ("error out"=w1256:errorcluster)  [unwired: 1 in, 9 out]
              }
            }
          }
          event "StopButton": Value Change {
            n351 = event-data() -> ()  [unwired: 2 out]
            n352 = Not(x=w1261) -> (.not. x?=w1260:bool)
          }
        }
        n353 = Not(x=w35) -> (.not. x?=w36:bool)
        n354 = call <vilib>:"Simple Error Handler.vi"("error in (no error)"=w28) -> ("error out"=w29:errorcluster)  [unwired: 1 in, 7 out]
        n355 = call <vilib>:"Clear Errors.vi"("error in (no error)"=w29) -> ("error out"=w30:errorcluster)  [unwired: 1 in, 5 out]
        "running" <- w35
      }
    }
    frame #2 {
      # "CLOSE"
      n356 = local read "OpenLED"() -> (w1264:bool)
      n357 = local write "running"(FALSE) -> ()
      n358 = case shown="True" w1264 {
        tunnel: w1263 -> [_ w1267]
        tunnel: w1262 -> [_ w1266]
        frame False {
        }
        frame True {
          n359 = call "MHM Close.vi"("error in (no error)"=w1267, "ulMHMHandle"=w1266) -> ()  [unwired: 8 in, 2 out]
        }
      }
    }
  }
  n360 = for {
    N: 4096 -> [_]
    tunnel: 4 ("x") -> [w1269]
    tunnel: [w1268] -> _ mode=indexing
    i -> [w1270]
    n361 = Multiply(x=w1269, y=w1270) -> (x*y=w1268:i32)
  }
